vi "Real Time_Master.vi"(4 "File Name":string="none", 8 "Ann Array Params":T1={"Synth Foc?"=FALSE, "Focal Zones"=41, "Switch T/R"=0, "Trans Geometry (mm)"={"Transducer"=0, "Geo Focus"=12.0, "a (radius)"=3.0, "# of rings"=5, "kerf space "=0.1, "Center Freq"=12.0}, "Sub Ap Excite?"=FALSE, "Full Array Scan?"=FALSE, "Xmt/Rcv"={"XMIT"=[TRUE, TRUE, TRUE, TRUE, TRUE], "RCV"=[TRUE, TRUE, TRUE, TRUE, TRUE]}, "PulseSpacing (us)"=0.0, "Xmit Ring"=0, "XMIT CHS"=0, "RCV CHS"=0, "GPU?"=FALSE, "Save TIFF?"=FALSE, "downfactor"=1, "RCV 1CH"=0} {"RCV 1CH" items=["All", "1", "2", "3", "4", "5"]; "Trans Geometry (mm)"."Transducer" items=["6D 12R 40 MHz"=0, "10D 31R 20 MHz"=1, "10D 23R 20 MHz"=2, "6D 23R 40 MHz"=3, "4.5D 10.7R 40 MHz"=4, "9D 23.5R 20 MHz"=5, "9D 25.8R 20MHz"=6, "Enter"=99]; "Switch T/R" min=1 max=5 step=1}, 10 "Motion Settings":T4={"No Motion?"=FALSE, "Motion System"=enum."NI 735x", "Motion Bd ID"=1, "Motion Profile"="SMAC1", "# Axis"=1, "Reverse Z axis?"=TRUE, "SMAC Axis"=0, "scan pair"=enum."y-(x) scan", "RT fps"=6.0, "Steps per mm"=[1000, 1000, 1000, 1000], "Motor Parameters"={"velocity ct/s"=[10000.0, 10000.0, 10000.0, 50000.0], "accel ct/s^2"=[50000.0, 50000.0, 50000.0, 200000.0]}, "One Way Scan"=FALSE, "Reverse One Way Scan"=FALSE, "Global Position (mm)"=[], "Plane"=0, "Distance between\nscan lines (um)"=0.0, "Distance between\nscan planes (um)"=0.0, "number of scan planes"=1, "Total steps in line"=0, "Xtra plane\ndistance  (um)"=100, "Xtra planes "=1, "Add Axis"=FALSE, "overshoot cts"=200, "BKPT Shift"=0, "Scan Start Time (ms)"=0, "ESP VISA"="GPIB::1::INSTR", "3rd Axis"=1, "GL Ref Out"=refnum, "Galil Address"=""} {"3rd Axis" items=["x", "y", "z", "w"]; "Xtra planes" min=1; "Xtra plane\ndistance  (um)" min=0; "Distance between\nscan planes (um)" format="%.2f"; "Distance between\nscan lines (um)" format="%.2f"; "SMAC Axis" items=["None"=0, "Axis 1"=1, "Axis 2"=2, "Axis 3"=3, "Axis 4"=4, "Axis 5"=5, "Axis 6"=6, "Axis 7"=7, "Axis 8"=8, "Vector Space 1"=17, "Vector Space 2"=18, "Vector Space 3"=19, "Vector Space 4"=20]; "Motion Bd ID" min=1 max=32 step=1}, 11 "Digitizer Settings":T8={"Digitizer delay (us) "=0.0, "rf points per line"=2048, "lines per plane"=128, "Samp Rate (Hz)"=100000000.0, "Additional dig delay (us)"=0.0, "Voltage Scale"=0.4, "Pre-Looks"=0, "Offset delay (us)"=0.0, "bits A/D"=8, "Avg Num"=1, "DigTimeOut"=5.0, "Rel Dig Delay"=0.0, "Dig Ch"=0, "LeCroyCluster"={"LeCroy Channels"=[TRUE, FALSE, FALSE, FALSE], "LC read pt offset"=0.0, "Sweep Avg"=FALSE}, "Main Digitizer"=enum."NI Digitizer", "Dig Config"=enum."Single channel", "Digitizer ID Cluster"={"Acqiris/Alazar/SP ID"=[], "NI Instr Handles"=[], "LeCroy VISA"="", "GaGe Handle"={"Handle"=0, "Sample size"=0, "Resolution"=0, "Offset"=0, "Channels"=0, "Boards"=0}, "ATS Ref"="ATS9350", "Acqiris Address"=["PCI::INSTR0"], "ADQRef"=refnum, "adq_cu_ptr"=refnum}, "Trigger Settings"={"Trig Source"=1, "Trig Coupling"=0, "Trig Slope"=0, "Level (mV)"=1500.0}, "Bulk Acq"=FALSE, "Bulk Start Indexes"=[], "Data Ref RF"=refnum, "NI ID/Channel"=[], "Total Dig CH"=1, "Xtra Ann Trig delay (us)"=10.0, "Fix Z Delay?"=FALSE, "One Way Transmission?"=FALSE, "Data Ref Log"=refnum} {"Trigger Settings"."Trig Slope" items=["Positive", "Negative"]; "Trigger Settings"."Level (mV)" format="%.2f"; "Trigger Settings"."Trig Coupling" items=["DC 1 MOhm", "AC 1 MOhm", "DC 50 Ohm", "AC 50 Ohm"]; "Trigger Settings"."Trig Source" items=["Chan 1", "External"]; "Rel Dig Delay" format="%.2f"; "DigTimeOut" format="%.2f"; "Avg Num" min=1; "Offset delay (us)" format="%.2f"; "Additional dig delay (us)" format="%.2f"; "Digitizer delay (us)" format="%.2f"}) -> (0 "Ann Array\nParams Out":T1={"Synth Foc?"=FALSE, "Focal Zones"=41, "Switch T/R"=0, "Trans Geometry (mm)"={"Transducer"=0, "Geo Focus"=12.0, "a (radius)"=3.0, "# of rings"=5, "kerf space "=0.1, "Center Freq"=12.0}, "Sub Ap Excite?"=FALSE, "Full Array Scan?"=FALSE, "Xmt/Rcv"={"XMIT"=[TRUE, TRUE, TRUE, TRUE, TRUE], "RCV"=[TRUE, TRUE, TRUE, TRUE, TRUE]}, "PulseSpacing (us)"=0.0, "Xmit Ring"=0, "XMIT CHS"=0, "RCV CHS"=0, "GPU?"=FALSE, "Save TIFF?"=FALSE, "downfactor"=1, "RCV 1CH"=0} {"RCV 1CH" items=["All", "1", "2", "3", "4", "5"]; "Trans Geometry (mm)"."Transducer" items=["6D 12R 40 MHz"=0, "10D 31R 20 MHz"=1, "10D 23R 20 MHz"=2, "6D 23R 40 MHz"=3, "4.5D 10.7R 40 MHz"=4, "9D 23.5R 20 MHz"=5, "9D 25.8R 20MHz"=6, "Enter"=99]; "Switch T/R" min=1 max=5 step=1}, 2 "Motion Settings Out":T4={"No Motion?"=FALSE, "Motion System"=enum."NI 735x", "Motion Bd ID"=1, "Motion Profile"="SMAC1", "# Axis"=1, "Reverse Z axis?"=TRUE, "SMAC Axis"=0, "scan pair"=enum."y-(x) scan", "RT fps"=6.0, "Steps per mm"=[1000, 1000, 1000, 1000], "Motor Parameters"={"velocity ct/s"=[10000.0, 10000.0, 10000.0, 50000.0], "accel ct/s^2"=[50000.0, 50000.0, 50000.0, 200000.0]}, "One Way Scan"=FALSE, "Reverse One Way Scan"=FALSE, "Global Position (mm)"=[], "Plane"=0, "Distance between\nscan lines (um)"=0.0, "Distance between\nscan planes (um)"=0.0, "number of scan planes"=1, "Total steps in line"=0, "Xtra plane\ndistance  (um)"=100, "Xtra planes "=1, "Add Axis"=FALSE, "overshoot cts"=200, "BKPT Shift"=0, "Scan Start Time (ms)"=0, "ESP VISA"="GPIB::1::INSTR", "3rd Axis"=1, "GL Ref Out"=refnum, "Galil Address"=""} {"3rd Axis" items=["x", "y", "z", "w"]; "Xtra planes" min=1; "Xtra plane\ndistance  (um)" min=0; "Distance between\nscan planes (um)" format="%.2f"; "Distance between\nscan lines (um)" format="%.2f"; "SMAC Axis" items=["None"=0, "Axis 1"=1, "Axis 2"=2, "Axis 3"=3, "Axis 4"=4, "Axis 5"=5, "Axis 6"=6, "Axis 7"=7, "Axis 8"=8, "Vector Space 1"=17, "Vector Space 2"=18, "Vector Space 3"=19, "Vector Space 4"=20]; "Motion Bd ID" min=1 max=32 step=1}, 3 "Digitizer Settings Out":T8={"Digitizer delay (us) "=0.0, "rf points per line"=2048, "lines per plane"=128, "Samp Rate (Hz)"=100000000.0, "Additional dig delay (us)"=0.0, "Voltage Scale"=0.4, "Pre-Looks"=0, "Offset delay (us)"=0.0, "bits A/D"=8, "Avg Num"=1, "DigTimeOut"=5.0, "Rel Dig Delay"=0.0, "Dig Ch"=0, "LeCroyCluster"={"LeCroy Channels"=[TRUE, FALSE, FALSE, FALSE], "LC read pt offset"=0.0, "Sweep Avg"=FALSE}, "Main Digitizer"=enum."NI Digitizer", "Dig Config"=enum."Single channel", "Digitizer ID Cluster"={"Acqiris/Alazar/SP ID"=[], "NI Instr Handles"=[], "LeCroy VISA"="", "GaGe Handle"={"Handle"=0, "Sample size"=0, "Resolution"=0, "Offset"=0, "Channels"=0, "Boards"=0}, "ATS Ref"="ATS9350", "Acqiris Address"=["PCI::INSTR0"], "ADQRef"=refnum, "adq_cu_ptr"=refnum}, "Trigger Settings"={"Trig Source"=1, "Trig Coupling"=0, "Trig Slope"=0, "Level (mV)"=1500.0}, "Bulk Acq"=FALSE, "Bulk Start Indexes"=[], "Data Ref RF"=refnum, "NI ID/Channel"=[], "Total Dig CH"=1, "Xtra Ann Trig delay (us)"=10.0, "Fix Z Delay?"=FALSE, "One Way Transmission?"=FALSE, "Data Ref Log"=refnum} {"Trigger Settings"."Trig Slope" items=["Positive", "Negative"]; "Trigger Settings"."Level (mV)" format="%.2f"; "Trigger Settings"."Trig Coupling" items=["DC 1 MOhm", "AC 1 MOhm", "DC 50 Ohm", "AC 50 Ohm"]; "Trigger Settings"."Trig Source" items=["Chan 1", "External"]; "Rel Dig Delay" format="%.2f"; "DigTimeOut" format="%.2f"; "Avg Num" min=1; "Offset delay (us)" format="%.2f"; "Additional dig delay (us)" format="%.2f"; "Digitizer delay (us)" format="%.2f"})   [LabVIEW 2022 SP3]
uses:
  ScanningControl/Digitizers/-DigitizerRoutines/DigitizerSettings.ctl
  ScanningControl/Digitizers/-DigitizerRoutines/Digitizer.ctl
  ScanningControl/Digitizers/-DigitizerRoutines/DigConfig.ctl
  ScanningControl/Digitizers/-DigitizerRoutines/DigitizerID.ctl
  C:/Windows/System32/ADQAPI_dotNet_helper.dll
  ScanningControl/Motion Controllers/NI_controller/-NI_MotionRoutines/MotionParameters.ctl
  ScanningControl/Motion Controllers/NI_controller/-NI_MotionRoutines/MotionSys.ctl
  ScanningControl/Motion Controllers/-MotionRoutines/ScanAxis.ctl
  ScanningControl/Motion Controllers/-MotionRoutines/3rdAxis.ctl
  Annular Array/-AnnularRoutines/TransGeometry.ctl
  Annular Array/-AnnularRoutines/ArrayGeometry.ctl
  Annular Array/-AnnularRoutines/AnnularArray.ctl
  <vilib>/Utility/miscctls.llb/LVRectTypeDef.ctl
  <vilib>/Utility/miscctls.llb/LVBoundsTypeDef.ctl
  <vilib>/picture/picture.llb/imagedata.ctl
  ScanningControl/Motion Controllers/Galil/Command Menu.ctl
  ScanningControl/Pulsers/PulserGlobals.vi
  ScanningControl/Motion Controllers/-MotionRoutines/MotionGlobals.vi
  <vilib>/Motion/FlexMotion/FunctionsVIs/Trajectory.llb/Load Acceleration/Deceleration.flx
  <vilib>/ptbypt/NI_PtbyPt.lvlib
  <vilib>/Motion/FlexMotion/FunctionsVIs/StartStopMotion.llb/Stop Motion (8 axes).flx
  <vilib>/Motion/FlexMotion/FunctionsVIs/StartStopMotion.llb/Start Motion (8 axes).flx
panel:
  in  "Flip X":bool
  out "No data":bool
  in  "options":T12(tab)
  in  "Focal Zones":i16=41
  in  "Trans Geometry (mm)":T2={"Transducer"=0, "Geo Focus"=12.0, "a (radius)"=3.0, "# of rings"=5, "kerf space "=0.1, "Center Freq"=12.0} {"Transducer" items=["6D 12R 40 MHz"=0, "10D 31R 20 MHz"=1, "10D 23R 20 MHz"=2, "6D 23R 40 MHz"=3, "4.5D 10.7R 40 MHz"=4, "9D 23.5R 20 MHz"=5, "9D 25.8R 20MHz"=6, "Enter"=99]}
  in  "Xmt/Rcv":cluster{"XMIT":bool[], "RCV":bool[]}={"XMIT"=[TRUE, TRUE, TRUE, TRUE, TRUE], "RCV"=[TRUE, TRUE, TRUE, TRUE, TRUE]}
  in  "GPU?":bool
  in  "Daxsonics Settings":T13={"Freq (MHz) "=20, "Amp (V)"=0, "Gain (dB)"=22} {"Freq (MHz)" items=["50"=20, "45"=27, "40"=34, "35"=41, "30"=49, "25"=56, "20"=63, "15"=70]; "Amp (V)" items=["100"=100, "90"=90, "80"=80, "70"=70, "60"=60, "50"=50, "40"=40, "30"=30, "20"=20, "10"=10, "0"=0]; "Gain (dB)" items=["64"=64, "60"=60, "52"=52, "48"=48, "44"=44, "40"=40, "36"=36, "32"=32, "28"=28, "24"=24, "20"=20, "16"=16]}
  in  "RF data Sampling":T14={"Sampling Rate"=100.0, "Ref Delay (ms)"=0.0, "rf points per line"=2048} {"rf points per line" min=1; "Ref Delay (ms)" format="%.2f"}
  in  "Voltage":dbl(ring)=0.2 items=["10 V"=10.0, "4 V"=4.0, "2 V"=2.0, "1 V"=1.0, "400 mV"=0.4, "200 mV"=0.2, "100 mV"=0.1]
  in  "Filter Prams":cluster{"low f":i32, "order":i32, "high F":i32}={"low f"=20, "order"=81, "high F"=65}
  in  "Filter":bool=TRUE
  in  "3D Acq":bool
  in  "Distance between\nplanes (mm)":i32=100 min=0
  in  "number of planes":u16=1
  out "Length of\nall planes (cm)":dbl=128.0 format="%.2f"
  in  "Axis":u16(ring)=1 items=["X Axis"=1, "Y Axis"=2, "Z Axis"=3, "W Axis"=4]
  in  "Position (mm) (Abs)":dbl format="%.3f"
  in  "Axis Tune":enum32{"Axis 1", "Axis 2", "Axis 3", "Axis 4"}(radio)=enum."Axis 2"
  in  "Stop Motor":bool
  in  "Adjust fps (%)":i16(slide)=100 min=0 max=150 scale=0.0..150.0
  in  "Accel":dbl(slide)=11928588.235294117 scale=1000000.0..6500000.0 scale format="%#_6e"
  in  "Inc. Step Size (mm)":dbl=0.5
  in  "LowTime":dbl=0.01
  in  "Gate Length":dbl=0.19 format="%.6f"
  in  "Xtra delay (us)":dbl=1.0
  in  "Aviso Sector":bool
  in  "Motion Parameters":T15={"lines per plane"=128, "Distance between\nscan lines (um)"=100.0, "Frames/s"=2.0, "BKPT Shift"=75, "Overshoot"=200} {"Overshoot" min=0 max=10000; "Distance between\nscan lines (um)" min=0.1 step=0.1; "lines per plane" min=1}
  out "Sat Ct":u8(slide) scale=0.0..400.0
  in  "Pause":bool
  in  "Center":bool
  in  "Scan":bool
  in  "Auto\nScale":bool
  in  "Save Raw":bool
  out "image time (ms)":u32
  out "Image Backlog":i32
  in  "Scale (dB)":cluster{i32, i32}(slide)={-55, 0} scale=0.0..-75.0
  in  "Fill":bool
  in  "1-to-1":bool
  out "InQueue":i32
  out "fps":dbl format="%#.2g"
  in  "N":u8=50 max=50 step=1
  in  "Save Last N EYE":bool
  out "Frame":i32
  in  "EYE CineLoop":bool
  in  "BMP CineLoop":bool
  out "Raw data":dbl[][](graph)
  in  "ExitSendCmd":bool
  # "View"
  # "Data Archiving"
  # "© 2011-2022 WCM"
  # "1-D and 2-D B scan settings"
  # "1-D and 2-D B scan settings"
  # "Daxsonics"
  # "Not working yet and slow."
  # "Cross Axis Motion"
  # "Scan"
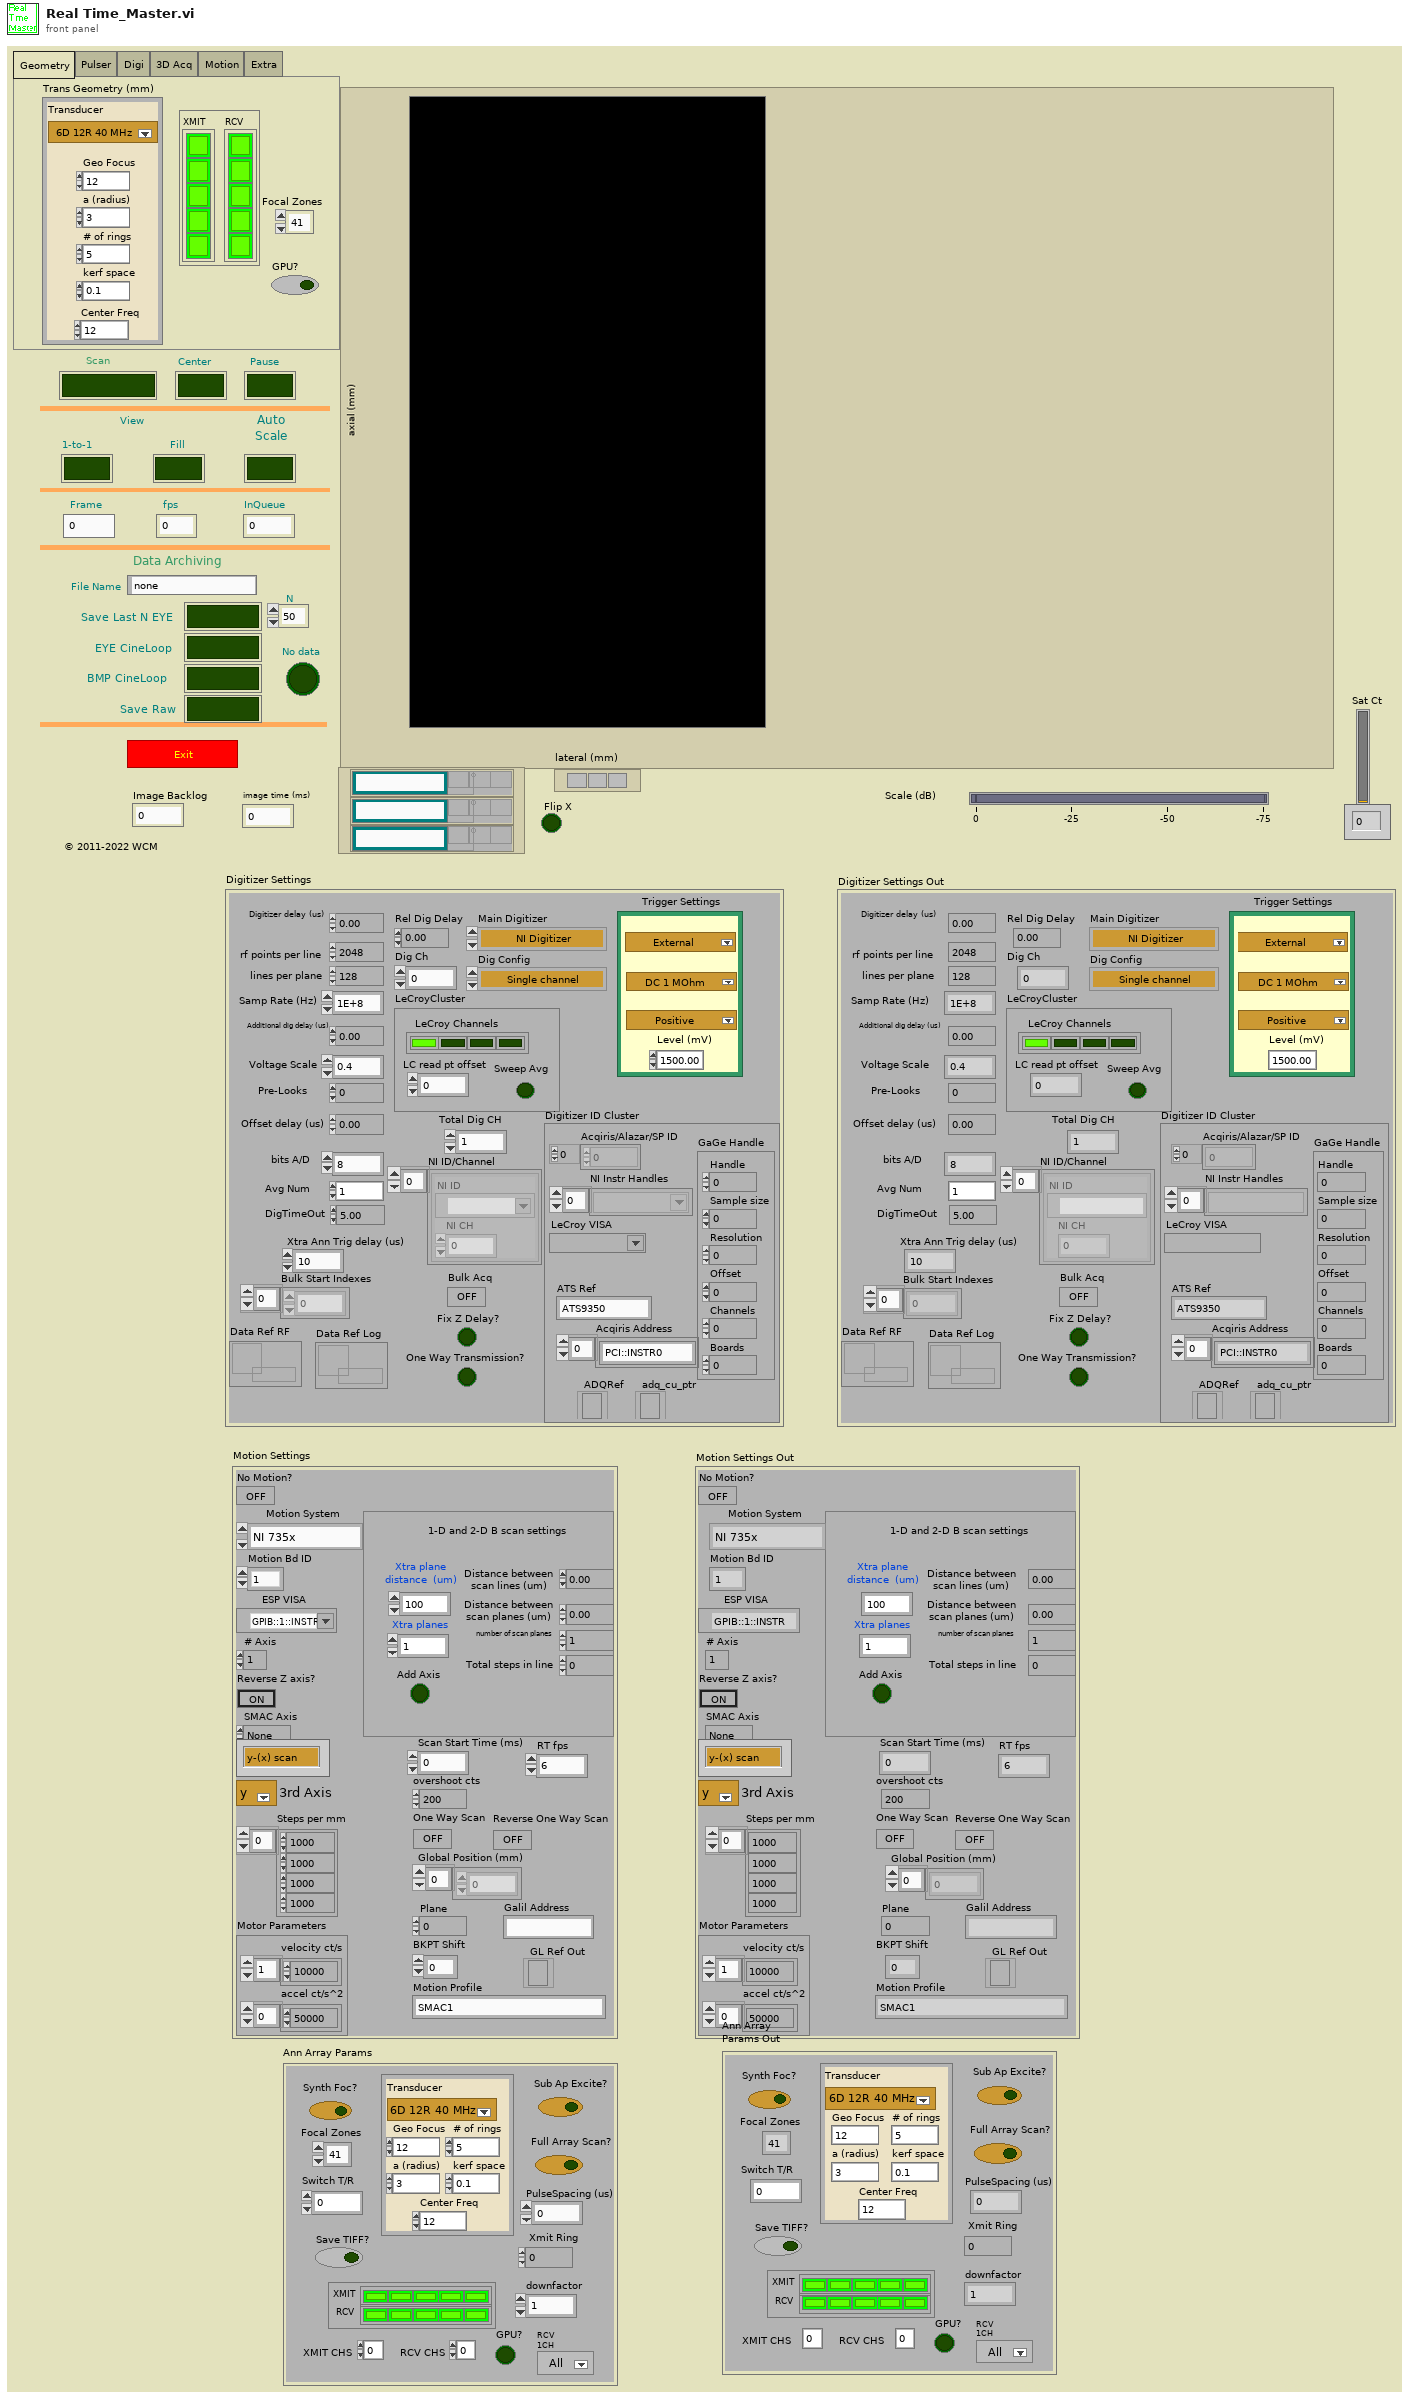
[diagram p1: front panel]
types:
  T1 = typedef "AnnularArray.ctl" = cluster{"Synth Foc?":bool, "Focal Zones":i16, "Switch T/R":i16, "Trans Geometry (mm)":T2, "Sub Ap Excite?":bool, "Full Array Scan?":bool, "Xmt/Rcv":cluster{"XMIT":bool[], "RCV":bool[]}, "PulseSpacing (us)":sgl, "Xmit Ring":i32, "XMIT CHS":u8, "RCV CHS":u8, "GPU?":bool, "Save TIFF?":bool, "downfactor":i32, "RCV 1CH":u16}
  T2 = typedef "TransGeometry.ctl" = cluster{"Transducer":T3, "Geo Focus":dbl, "a (radius)":dbl, "# of rings":i32, "kerf space ":dbl, "Center Freq":dbl}
  T3 = typedef "ArrayGeometry.ctl" = u16
  T4 = typedef "MotionParameters.ctl" = cluster{"No Motion?":bool, "Motion System":T5, "Motion Bd ID":u8, "Motion Profile":string, "# Axis":i8, "Reverse Z axis?":bool, "SMAC Axis":u16, "scan pair":T6, "RT fps":sgl, "Steps per mm":i32[], "Motor Parameters":cluster{"velocity ct/s":dbl[], "accel ct/s^2":dbl[]}, "One Way Scan":bool, "Reverse One Way Scan":bool, "Global Position (mm)":dbl[], "Plane":i32, "Distance between\nscan lines (um)":sgl, "Distance between\nscan planes (um)":sgl, "number of scan planes":i32, "Total steps in line":i32, "Xtra plane\ndistance  (um)":i32, "Xtra planes ":i32, "Add Axis":bool, "overshoot cts":i32, "BKPT Shift":i32, "Scan Start Time (ms)":u32, "ESP VISA":refnum<visa-resource-name>, "3rd Axis":T7, "GL Ref Out":refnum<k7>, "Galil Address":string}
  T5 = typedef "MotionSys.ctl" = enum16{"MM3000", "NI 735x", "Newport ESP", "No Motion Card", "Galil"}
  T6 = typedef "ScanAxis.ctl" = enum16{"y-(x) scan", "x-(y) scan", "z-(x) scan", "z-(y) scan", "y-(z) scan", "x-(z) scan", "w-(x) scan", "w-(y) scan", "w-(z) scan", "x-(w) scan", "y-(w) scan", "z-(w) scan"}
  T7 = typedef "3rdAxis.ctl" = u16
  T8 = typedef "DigitizerSettings.ctl" = cluster{"Digitizer delay (us) ":dbl, "rf points per line":i32, "lines per plane":i32, "Samp Rate (Hz)":dbl, "Additional dig delay (us)":dbl, "Voltage Scale":dbl, "Pre-Looks":i32, "Offset delay (us)":dbl, "bits A/D":i8, "Avg Num":i32, "DigTimeOut":sgl, "Rel Dig Delay":sgl, "Dig Ch":i32, "LeCroyCluster":cluster{"LeCroy Channels":bool[], "LC read pt offset":dbl, "Sweep Avg":bool}, "Main Digitizer":T9, "Dig Config":T10, "Digitizer ID Cluster":T11, "Trigger Settings":cluster{"Trig Source":u16, "Trig Coupling":u16, "Trig Slope":u16, "Level (mV)":dbl}, "Bulk Acq":bool, "Bulk Start Indexes":i32[], "Data Ref RF":refnum<data-value>, "NI ID/Channel":cluster{"NI ID":refnum<k15>, "NI CH":i32}[], "Total Dig CH":i32, "Xtra Ann Trig delay (us)":dbl, "Fix Z Delay?":bool, "One Way Transmission?":bool, "Data Ref Log":refnum<data-value>}
  T9 = typedef "Digitizer.ctl" = enum16{"Acqiris Digitizer", "NI Digitizer", "LeCroy", "GaGe", "AlazarTech", "No Digitizer", "Teledyne"}
  T10 = typedef "DigConfig.ctl" = enum16{"Single channel", "2 Chans w/ 2 Acqiris", "2 Chans w/ 1 Acqiris", "5-CH Pulser New", "5-CH pulser w/ ann array", "5-pass style ann array", "Empty"}
  T11 = typedef "DigitizerID.ctl" = cluster{"Acqiris/Alazar/SP ID":u32[], "NI Instr Handles":refnum<k15>[], "LeCroy VISA":refnum<visa-resource-name>, "GaGe Handle":cluster{"Handle":u32, "Sample size":u32, "Resolution":i32, "Offset":i32, "Channels":u32, "Boards":u32}, "ATS Ref":string, "Acqiris Address":string[], "ADQRef":refnum<k24>, "adq_cu_ptr":refnum<k24>}
  T12 = enum32{"Geometry", "Pulser", "Digi", "3D Acq", "Motion", "Extra"}
  T13 = cluster{"Freq (MHz) ":u16, "Amp (V)":u16, "Gain (dB)":u16}
  T14 = cluster{"Sampling Rate":dbl, "Ref Delay (ms)":dbl, "rf points per line":i32}
  T15 = cluster{"lines per plane":u16, "Distance between\nscan lines (um)":sgl, "Frames/s":sgl, "BKPT Shift":i32, "Overshoot":i32}
  T16 = typedef "LVBoundsTypeDef.ctl" = cluster{"Width":u32, "Height":u32}
  T17 = typedef "LVRectTypeDef.ctl" = cluster{"Left":i16, "Top":i16, "Right":i16, "Bottom":i16}
  T18 = typedef "pulser.ctl" = enum16{"Pan 5900", "Daxsonics", "Agilent 33xxx", "UTEX", "JSR", "WMC Mono-Cycle", "No Pulser", "NYU AVTECH", "Tabor W1281A", "Pan 5800", "Unlisted", "Tabor WX2182B"}
  T19 = typedef "location.ctl" = enum16{"Automatic", "WCM Main", "Hawaii", "Columbia MM3000", "Columbia  NI System", "NYU", "RRI 2", "UHI Allen", "CUMC RT", "Chiba", "Stony Brook", "WCM Microscopy", "WCM Aeoretch", "WCM Optics Lab", "WCM Main 2Axis", "WCM Rotation", "WCM SAM SMAC", "SERI GP"}
  T20 = cluster{"DataBufferQ":refnum<queue>, "LastNQ":refnum<queue>, "LastNBMPQ":refnum<queue>, "SaveRawN":refnum<notifier>, "StopN":refnum<notifier>}
  T21 = typedef "imagedata.ctl" = cluster{"image type":i32, "image depth":i32, "image":u8[], "mask":u8[], "colors":u32[], "Rectangle":cluster{"left":i16, "top":i16, "right":i16, "bottom":i16}}
  T22 = cluster{"gain":dbl, bool, "wfm":i16[][], i32, bool}
  T23 = enum16{"Absolute Position", "Relative Position", "Velocity", "Relative to Cap Pos", "Modulus Position", "Absolute Contouring", "Relative Contouring"}
  T24 = cluster{"Voltage Scale":dbl, "Offset":dbl, "Coupling":u16}
  T25 = enum16{"Home", "Index", "Center", "Forward Limit", "Reverse Limit", "Run Sequence"}
  T26 = typedef "Command Menu.ctl" = enum16{"CommandPassThrough", "Abort Motion", "Define Pos", "Velocity", "Acceleration", "Deceleration", "Position Rel", "Postion Abs", "Begin Move", "After Move", "Home", "KI", "KD", "KP", "IL", "Config I/O", "Set Bit", "Clear Bit", "Motor Off", "Moto On", "Status", "Execute", "Halt Execute", "HX Status", "Tell Velocity", "Check Motion", "BreakPoint", "Tell Position", "Current Code Line", "Tell Switches", "OC Force On", "OC Off", "Pos Soft Limit", "Rev Soft Limit"}
  T27 = typedef "LVStringsAndValuesArrayTypeDef_DBL.ctl" = cluster{"String":string, "Value":dbl}[]
  T28 = cluster{"Samp Rate (Hz)":dbl, "Digitizer delay (us) ":dbl, "rf points per line":i32}
  T29 = typedef "LVStringsAndValuesArrayTypeDef_U16.ctl" = cluster{"String":string, "Value":u16}[]
  T30 = typedef "Dax_Control_Cluster.ctl" = cluster{"Freq (MHz) ":u16, "Voltage (V)":u16, "Gain (dB)":u16}
  T31 = cluster{"Axis scaling Params":cluster{"X right":dbl, "X left":dbl, "Y low":dbl, "Y high":dbl}, "x scaled":dbl[][], "y scaled":dbl[][], "scales":cluster{"inc x (mm)":dbl, "inc y (mm)":dbl}, "Array":dbl[][], "pixels in x":i16, "pixels in y":i16}
  T32 = cluster{"FIR Windowed Coefficients":dbl[], "Filter Prams":cluster{"low f":i32, "order":i32, "high F":i32}}
  T33 = cluster{"gain":dbl, bool, "wfm":i16[][], "max queue size (-1, unlimited)":i32, "Time Out":bool}
  T34 = typedef "eventvkey.ctl" = enum16{"ASCII", "Enter", "Return", "Shift", "Ctrl", "Alt", "Cmd", "Opt", "Caps", "NumLock", "Clear", "Break", "Up", "Down", "Left", "Right", "Insert", "Delete", "Home", "End", "PageUp", "PageDown", "Escape", "Help", "Pause", "ScrollLock", "F1", "F2", "F3", "F4", "F5", "F6", "F7", "F8", "F9", "F10", "F11", "F12", "F13", "F14", "F15", "F16", "F17", "F18", "F19", "F20", "F21", "F22", "F23", "F24", "Play", "VolumeUp", "VolumeDown", "Mute", "Two Byte Char"}
  T35 = cluster{"Shift":bool, "Ctrl":bool, "Alt":bool, "Cmd":bool, "Opt":bool}
  T36 = typedef "Resource Out (Enum).flx" = u16
  T37 = typedef "Bd Id Out" = u8
  T38 = cluster{"Y Scale Offset":dbl, "Y Scale Multi":dbl, "X Scale Offset":dbl, "X Scale Multi":dbl, "Gate Distance":dbl}
  T39 = typedef "AxisOrVectorSpaceControl To Control.flx" = u16
  T40 = typedef "LVRangeTypeDef.ctl" = cluster{"Minimum":dbl, "Maximum":dbl, "Increment":dbl, "Minor Increment":dbl, "Start":dbl}
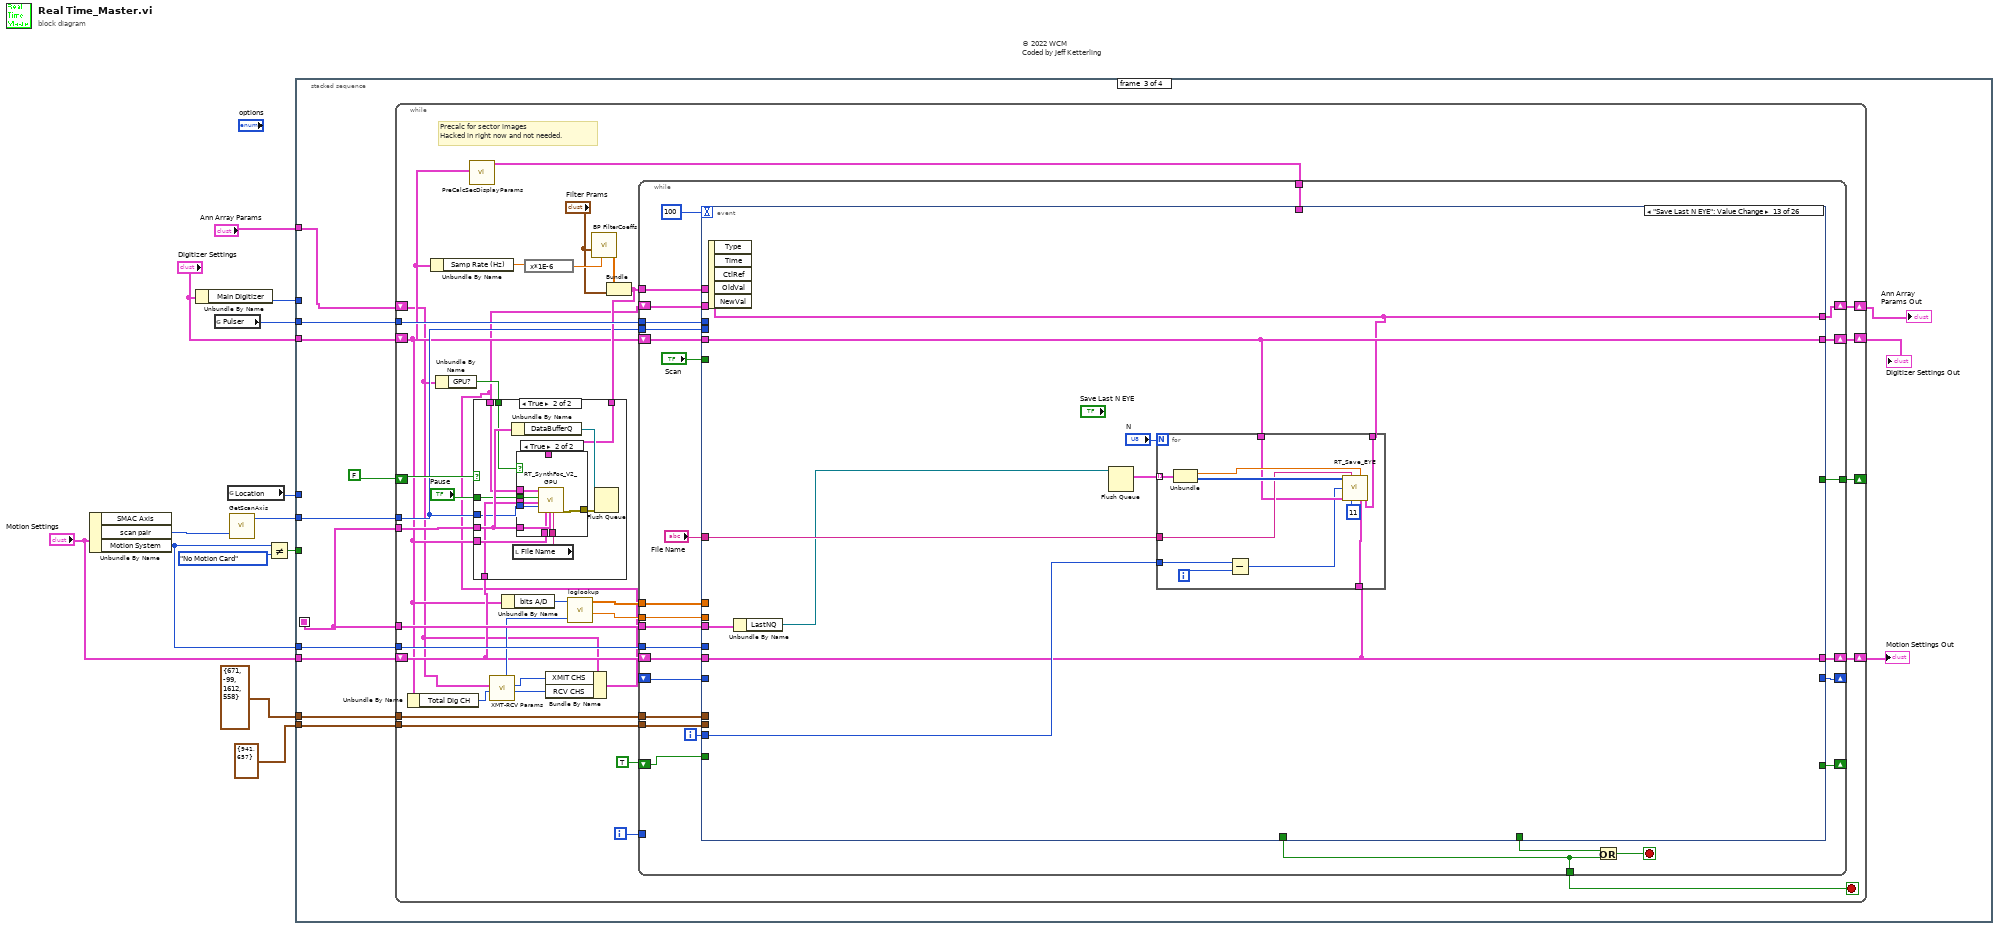
[diagram p0: block diagram]
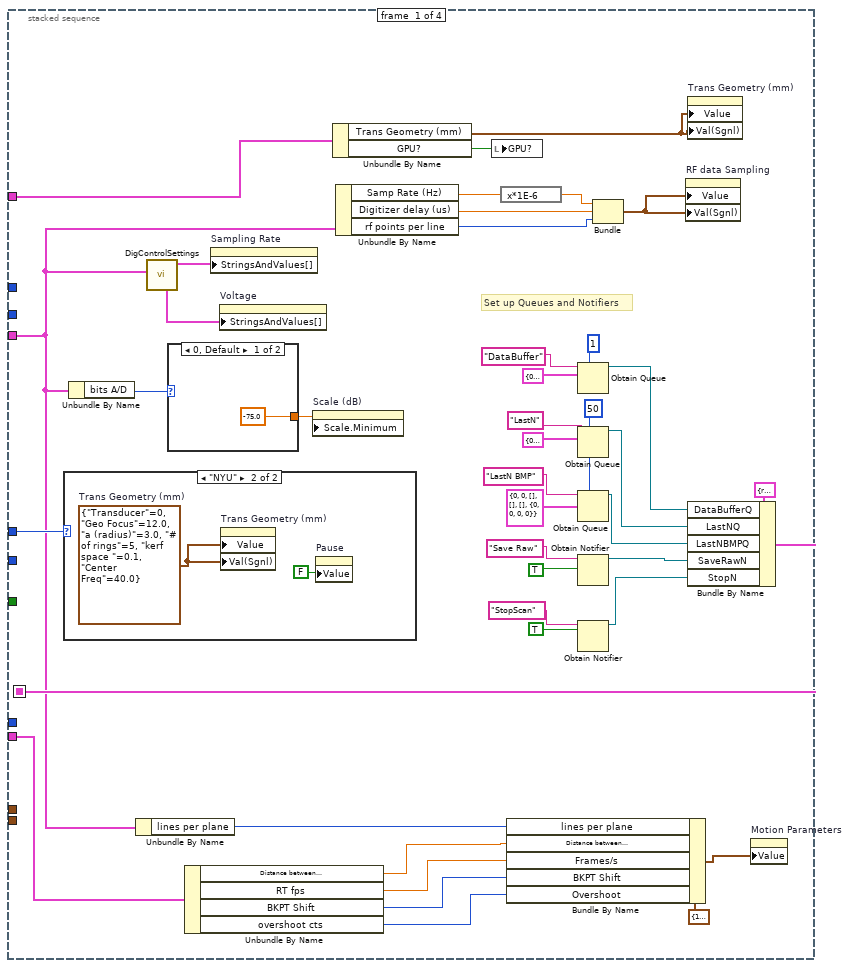
[diagram p2: hidden frame]
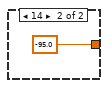
[diagram p4: hidden frame]
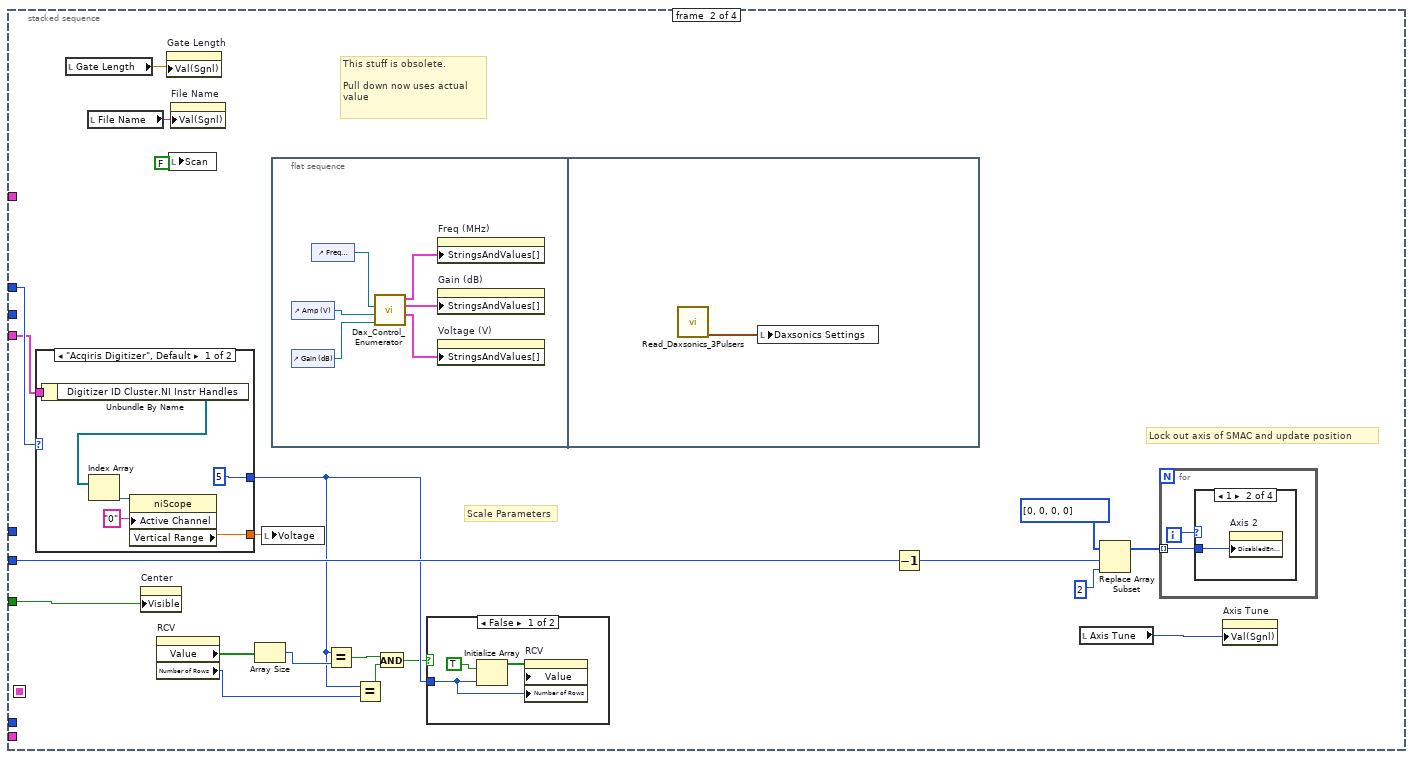
[diagram p5: hidden frame]
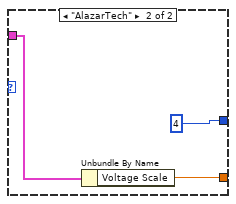
[diagram p7: hidden frame]
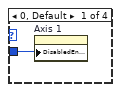
[diagram p8: hidden frame]
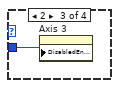
[diagram p9: hidden frame]
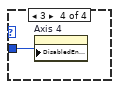
[diagram p10: hidden frame]
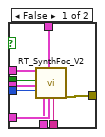
[diagram p12: hidden frame]
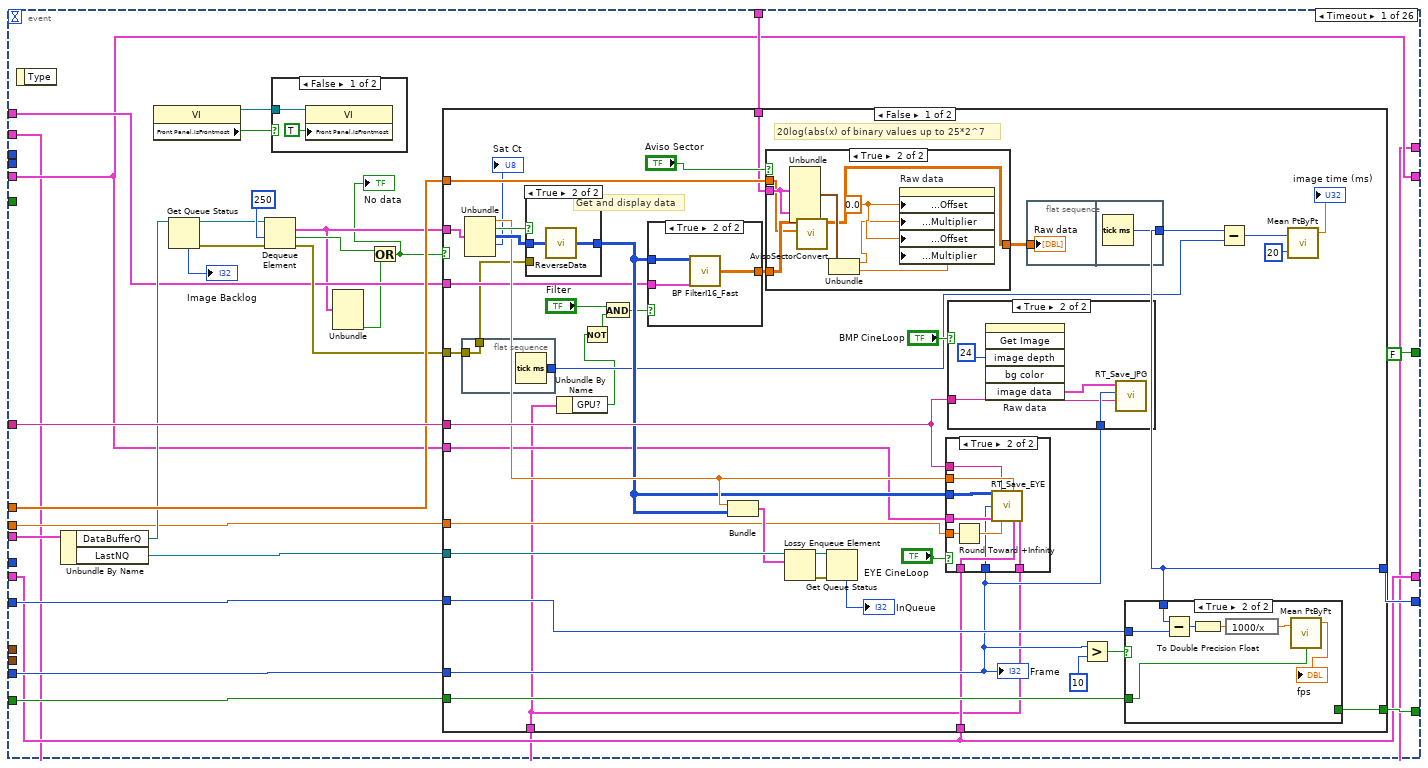
[diagram p13: hidden frame]
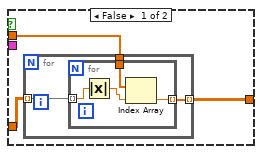
[diagram p15: hidden frame]
diagram:
  # "© 2022 WCM\nCoded by Jeff Ketterling"
  n1 = Unbundle By Name("Motion Settings") -> ("scan pair"=w6:T6, "Motion System"=w7:T5)  [unwired: 1 out]
  n2 = Unbundle By Name("Digitizer Settings") -> ("Main Digitizer"=w9:T9)
  n3 = global read "PulserGlobals.vi" "Pulser"() -> (w4:T18)
  n4 = global read "MotionGlobals.vi" "Location"() -> (w2:T19)
  n5 = call "GetScanAxis.vi"("scan pair"=w6) -> ("Axis 1"=w5:i32)  [unwired: 1 in, 2 out]
  n6 = Not Equal?(x=w7, y=MotionSys."No Motion Card" ("Motion System")) -> (x != y?=w11:bool)
  n7 = stacked-sequence {
    seq-local: [w38 _ _ _] -> [_ _ w112 w857]
    tunnel: T16 {"Width"=941, "Height"=657} ("Plot Area:Size") -> [_ _ w115 _]
    tunnel: T17 {"Left"=671, "Top"=-99, "Right"=1612, "Bottom"=558} ("Plot Area Bounds") -> [_ _ w114 _]
    tunnel: w5 -> [_ w72 w113 _]
    tunnel: w11 -> [_ w76 _ _]
    tunnel: w7 -> [_ _ w111 _]
    tunnel: w4 -> [_ _ w110 _]
    tunnel: w9 -> [_ w68 _ _]
    tunnel: "Digitizer Settings" -> [w14 w59 w109 _]
    tunnel: "Motion Settings" -> [w23 _ w107 _]
    tunnel: w2 -> [w26 _ _ _]
    tunnel: "Ann Array Params" -> [w24 _ w104 _]
    frame #0 {
      w31 = 50 ("max queue size (-1, unlimited)")
      # "Set up Queues and Notifiers"
      n8 = case shown="\"NYU\"" w26 {
        frame "WCM Main", Default {
        }
        frame "NYU" {
          w55 = T2 {"Transducer"=0, "Geo Focus"=12.0, "a (radius)"=3.0, "# of rings"=5, "kerf space "=0.1, "Center Freq"=40.0}  # Trans Geometry (mm)
          n9 = property on="Trans Geometry (mm)" class="Clust (strict)"("Value"=w55, "Val(Sgnl)"=w55) -> ()  [unwired: 2 in, 2 out]
          n10 = property on="Pause" class="Bool (strict)"("Value"=FALSE ("Pause")) -> ()  [unwired: 2 in, 2 out]
        }
      }
      n11 = Unbundle By Name(w14) -> ("bits A/D"=w27:i8)
      n12 = Unbundle By Name(w14) -> ("lines per plane"=w22:i32)
      n13 = call "DigControlSettings.vi"("Digitizer Settings"=w14) -> ("Sampling Rates"=w34:T27, "Voltage Scale"=w33:T27)  [unwired: 6 in, 3 out]
      n14 = case shown="0, Default" w27 {
        tunnel: [-75.0 ("Scale.Range:Maximum") -95.0 ("Scale.Range:Maximum")] -> w32
        frame 0, Default {
        }
        frame 14 {
        }
      }
      n15 = Unbundle By Name(w23) -> ("Distance between\nscan lines (um)"=w21:sgl, "RT fps"=w20:sgl, "BKPT Shift"=w19:i32, "overshoot cts"=w18:i32)
      n16 = property on="Sampling Rate" class="Ring (strict)"("StringsAndValues[]"=w34) -> ()  [unwired: 2 in, 2 out]
      n17 = property on="Voltage" class="Ring (strict)"("StringsAndValues[]"=w33) -> ()  [unwired: 2 in, 2 out]
      n18 = property on="Scale (dB)" class="Slide (strict)"("Scale.Minimum"=w32) -> ()  [unwired: 2 in, 2 out]
      n19 = Unbundle By Name(w24) -> ("Trans Geometry (mm)"=w15:T2, "GPU?"=w25:bool)
      n20 = Unbundle By Name(w14) -> ("Samp Rate (Hz)"=w30:dbl, "Digitizer delay (us)"=w29:dbl, "rf points per line"=w28:i32)
      n21 = local write "GPU?"(w25) -> ()
      n22 = expression code="x*1E-6"(w30) -> (w35:dbl)
      n23 = Bundle By Name(cluster=T15 {"lines per plane"=128, "Distance between\nscan lines (um)"=100.0, "Frames/s"=2.0, "BKPT Shift"=75, "Overshoot"=200} ("Motion Parameters"), "lines per plane"=w22, "Distance between\nscan lines (um)"=w21, "Frames/s"=w20, "BKPT Shift"=w19, "Overshoot"=w18) -> (w16:T15)
      n24 = Obtain Queue(max queue size (-1, unlimited)=1, name (unnamed)="DataBuffer", element data type=T22 {"gain"=0.0, TRUE, "wfm"=[], 0, TRUE}) -> (queue out=w41:refnum<queue>)  [unwired: 2 in, 2 out]
      n25 = Obtain Queue ("LastN")(max queue size (-1, unlimited)=w31, name (unnamed)="LastN", element data type=cluster{"gain":dbl, "wfm":i16[][]} {"gain"=0.0, "wfm"=[]}) -> (queue out=w42:refnum<queue>)  [unwired: 2 in, 2 out]
      n26 = Obtain Queue ("LastNBMP")(max queue size (-1, unlimited)=w31, name (unnamed)="LastN BMP", element data type=T21 {"image type"=0, "image depth"=0, "image"=[], "mask"=[], "colors"=[], "Rectangle"={"left"=0, "top"=0, "right"=0, "bottom"=0}} ("Image Data")) -> (queue out=w40:refnum<queue>)  [unwired: 2 in, 2 out]
      n27 = Obtain Notifier ("Raw eye")(name (unnamed)="Save Raw", notification data type=TRUE) -> (notifier out=w43:refnum<notifier>)  [unwired: 2 in, 2 out]
      n28 = Obtain Notifier ("Stop Scan")(name (unnamed)="StopScan", notification data type=TRUE) -> (notifier out=w39:refnum<notifier>)  [unwired: 2 in, 2 out]
      n29 = Bundle("Samp Rate (Hz)"=w35, "Digitizer delay (us)"=w29, "rf points per line"=w28) -> (w36:T28)  [unwired: 1 in]
      n30 = property on="RF data Sampling" class="Clust (strict)"("Value"=w36, "Val(Sgnl)"=w36) -> ()  [unwired: 2 in, 2 out]
      n31 = property on="Trans Geometry (mm)" class="Clust (strict)"("Value"=w15, "Val(Sgnl)"=w15) -> ()  [unwired: 2 in, 2 out]
      n32 = Bundle By Name(cluster=T20 {"DataBufferQ"=refnum, "LastNQ"=refnum, "LastNBMPQ"=refnum, "SaveRawN"=refnum, "StopN"=refnum} ("Qs and Notis"), "DataBufferQ"=w41, "LastNQ"=w42, "LastNBMPQ"=w40, "SaveRawN"=w43, "StopN"=w39) -> (w38:T20)
      n33 = property on="Motion Parameters" class="Clust (strict)"("Value"=w16) -> ()  [unwired: 2 in, 2 out]
    }
    frame #1 {
      # "This stuff is obsolete.\n\nPull down now uses actual value"
      # "Lock out axis of SMAC and update position"
      # "Scale Parameters"
      n34 = case shown="\"Acqiris Digitizer\", Default" w68 {
        tunnel: [w85 w88] -> w69
        tunnel: [5 4] -> w65
        tunnel: w59 -> [w82 w89]
        frame "Acqiris Digitizer", Default {
          n35 = Unbundle By Name(w82) -> ("Digitizer ID Cluster.NI Instr Handles"=w83:refnum<k15>[])
          n36 = Index Array(array=w83) -> (element=w87:refnum<k15>)  [unwired: 1 in]
          n37 = property class="niScope"(reference=w87, "Active Channel"="0") -> ("Vertical Range"=w85:dbl)  [unwired: 1 in, 2 out]
        }
        frame "AlazarTech" {
          n38 = Unbundle By Name(w89) -> ("Voltage Scale"=w88:dbl)
        }
      }
      n39 = local read "Gate Length"() -> (w60:dbl)
      n40 = local read "File Name"() -> (w77:string)
      n41 = property on="Center" class="Bool"("Visible"=w76) -> ()  [unwired: 2 in, 2 out]
      n42 = property on="RCV" class="Arr (strict)"() -> ("Value"=w67:bool[], "Number of Rows"=w64:u32)  [unwired: 2 in, 2 out]
      n43 = property on="Gate Length" class="DigNum (strict)"("Val(Sgnl)"=w60) -> ()  [unwired: 2 in, 2 out]
      n44 = local write "Scan"(FALSE ("go")) -> ()
      n45 = property on="File Name" class="Str"("Val(Sgnl)"=w77) -> ()  [unwired: 2 in, 2 out]
      n46 = Array Size(array=w67) -> (size(s)=w66:i32)
      n47 = local write "Voltage"(w69) -> ()
      n48 = flat-sequence {
        frame #0 {
          n49 = control-ref of="Amp (V)"() -> (w92:refnum<vi>)
          n50 = control-ref of="Gain (dB)"() -> (w91:refnum<vi>)
          n51 = control-ref of="Freq (MHz)"() -> (w93:refnum<vi>)
          n52 = call "Dax_Control_Enumerator.vi"("Gain (dB) Ref"=w91, "Voltage (V) Ref"=w92, "Freq (MHz) Ref"=w93) -> ("Voltage"=w94:T29, "Gain"=w95:T29, "Freq"=w96:T29)  [unwired: 6 in]
          n53 = property on="Freq (MHz)" class="Ring (strict)"("StringsAndValues[]"=w96) -> ()  [unwired: 2 in, 2 out]
          n54 = property on="Gain (dB)" class="Ring (strict)"("StringsAndValues[]"=w95) -> ()  [unwired: 2 in, 2 out]
          n55 = property on="Voltage (V)" class="Ring (strict)"("StringsAndValues[]"=w94) -> ()  [unwired: 2 in, 2 out]
        }
        frame #1 {
          n56 = call "Read_Daxsonics_3Pulsers.vi"() -> ("Dax Values"=w97:T30)  [unwired: 5 in, 6 out]
          n57 = local write "Daxsonics Settings"(w97) -> ()
        }
      }
      n58 = Equal?(x=w65, y=w66) -> (x = y?=w63:bool)
      n59 = Equal?(x=w65, y=w64) -> (x = y?=w62:bool)
      n60 = And(x=w63, y=w62) -> (x .and. y?=w61:bool)
      n61 = case shown="False" w61 {
        tunnel: w65 -> [w79 _]
        frame False {
          n62 = Initialize Array(TRUE, w79) -> (w80:bool[])
          n63 = property on="RCV" class="Arr (strict)"("Value"=w80, "Number of Rows"=w79) -> ()  [unwired: 2 in, 2 out]
        }
        frame True {
        }
      }
      n64 = Decrement(x=w72) -> (x-1=w70:i32)
      n65 = local read "Axis Tune"() -> (w71:enum32{"Axis 1", "Axis 2", "Axis 3", "Axis 4"})
      n66 = Replace Array Subset(array=i32[] [0, 0, 0, 0], new element=2 ("new element/subarray"), index=w70) -> (w73:i32[])
      n67 = for {
        tunnel: w73 -> [w98] mode=indexing
        i -> [w99]
        n68 = case shown="1" w99 {
          tunnel: w98 -> [w100 w101 w102 w103]
          frame 0, Default {
            n69 = property on="Axis 1" class="Bool (strict)"("DisabledEnum"=w100) -> ()  [unwired: 2 in, 2 out]
          }
          frame 1 {
            n70 = property on="Axis 2" class="Bool (strict)"("DisabledEnum"=w101) -> ()  [unwired: 2 in, 2 out]
          }
          frame 2 {
            n71 = property on="Axis 3" class="Bool (strict)"("DisabledEnum"=w102) -> ()  [unwired: 2 in, 2 out]
          }
          frame 3 {
            n72 = property on="Axis 4" class="Bool (strict)"("DisabledEnum"=w103) -> ()  [unwired: 2 in, 2 out]
          }
        }
      }
      n73 = property on="Axis Tune" class="RadioBtnsControl (strict)"("Val(Sgnl)"=w71) -> ()  [unwired: 2 in, 2 out]
    }
    frame #2 {
      n74 = while {
        shift-right: [w149] -> _
        shift-left: FALSE ("go") -> [w150]
        tunnel: w115 -> [w146]
        tunnel: w114 -> [w145]
        tunnel: w113 -> [w125]
        tunnel: w112 -> [w142]
        tunnel: w112 -> [w141]
        tunnel: w111 -> [w138]
        tunnel: w110 -> [w137]
        shift-right: [w130] -> w108
        shift-left: w109 -> [w124]
        shift-right: [w126] -> w106
        shift-left: w107 -> [w127]
        shift-right: [w120] -> w105
        shift-left: w104 -> [w118]
        i -> [w147]
        stop <- w148 stop-if-true
        # "Precalc for sector images\nHacked in right now and not needed."
        n75 = Unbundle By Name(w124) -> ("Total Dig CH"=w123:i32)
        n76 = Unbundle By Name(w124) -> ("Samp Rate (Hz)"=w131:dbl)
        n77 = Unbundle By Name(w118) -> ("GPU?"=w119:bool)
        n78 = call "PreCalcSecDisplayParams.vi"("Digitizer Settings"=w124) -> ("Cluster out"=w128:T31)  [unwired: 10 in]
        n79 = call "XMT-RCV Params.vi"("Dig Channels"=w123, "Ann Array Params"=w118) -> ("# RCV"=w121:i16, "# XMIT"=w122:i16, "virtual T/R count"=w133:i16)  [unwired: 4 in, 3 out]
        n80 = Unbundle By Name(w124) -> ("bits A/D"=w129:i8)
        n81 = expression code="x*1E-6"(w131) -> (w140:dbl)
        n82 = Bundle By Name(cluster=w118, "XMIT CHS"=w122, "RCV CHS"=w121) -> (w117:T1)
        n83 = call "loglookup.vi"("A/D bits"=w129, "virtual T/R Pairs"=w133) -> ("Log Lookup"=w143:sgl[], "BFormed Bits"=w132:dbl)  [unwired: 1 in, 2 out]
        n84 = call "BP FilterCoeffs.vi"("sample rate MHz"=w140, "Filter Prams"="Filter Prams") -> ("FIR Windowed Coefficients"=w136:dbl[])  [unwired: 4 in]
        n85 = Bundle("FIR Windowed Coefficients"=w136, "Filter Prams"="Filter Prams") -> (w134:T32)  [unwired: 1 in]
        n86 = case shown="True" w150 {
          tunnel: w142 -> [_ w160]
          tunnel: "Pause" -> [_ w157]
          tunnel: w134 -> [_ w156]
          tunnel: w124 -> [_ w155]
          tunnel: w127 -> [_ w154]
          tunnel: w125 -> [_ w153]
          tunnel: w117 -> [_ w152]
          tunnel: w119 -> [_ w151]
          frame False {
          }
          frame True {
            n87 = Unbundle By Name(w160) -> ("DataBufferQ"=w159:refnum<queue>)
            n88 = local read "File Name"() -> (w158:string)
            n89 = case shown="True" w151 {
              tunnel: [w170 w178] -> w161
              tunnel: w160 -> [w169 w177]
              tunnel: w158 -> [w168 w176]
              tunnel: w157 -> [w167 w175]
              tunnel: w156 -> [w166 _]
              tunnel: w155 -> [w165 w174]
              tunnel: w154 -> [w164 w173]
              tunnel: w153 -> [w163 w172]
              tunnel: w152 -> [w162 w171]
              frame False {
                n90 = call "RT_SynthFoc_V2.vi"("Ann Array Params"=w162, "Pause?"=w167, "Motion Settings"=w164, "Scan Axis"=w163, "Digitizer Settings"=w165, "Filter"=w166, "Qs and Notis"=w169, "Raw Name"=w168) -> ("error out"=w170:errorcluster)  [unwired: 10 in, 1 out]
              }
              frame True {
                n91 = call "RT_SynthFoc_V2_GPU.vi"("Ann Array Params"=w171, "Pause?"=w175, "Motion Settings"=w173, "Scan Axis"=w172, "Digitizer Settings"=w174, "Qs and Notis"=w177, "Raw Name"=w176) -> ("error out"=w178:errorcluster)  [unwired: 11 in, 1 out]
              }
            }
            n92 = Flush Queue(queue=w159, error in (no error)=w161) -> ()  [unwired: 3 out]
          }
        }
        n93 = while {
          tunnel: [w203] -> w149
          tunnel: [w200] -> w148
          tunnel: w147 -> [_]
          shift-right: [w199] -> _
          shift-left: _ -> [w198]
          tunnel: w146 -> [w197]
          tunnel: w145 -> [w196]
          tunnel: w125 -> [w195]
          shift-right: [w193] -> _
          shift-left: TRUE -> [w194]
          tunnel: w143 -> [w192]
          tunnel: w141 -> [w190]
          tunnel: w138 -> [w189]
          tunnel: w137 -> [w188]
          tunnel: w134 -> [w187]
          tunnel: w132 -> [w186]
          tunnel: w128 -> [w185]
          shift-right: [w183] -> w130
          shift-left: w124 -> [w184]
          shift-right: [w181] -> w126
          shift-left: w127 -> [w182]
          shift-right: [w179] -> w120
          shift-left: w117 -> [w180]
          i -> [w206]
          stop <- w201 stop-if-true
          n94 = event shown="[12] \"Save Last N EYE\": Value Change" {
            selector: _ -> [_ _ _ _ _ _ _ _ _ _ _ _ _ _ _ _ _ _ _ _ _ _ _ _ _ _]
            dyn-events: _ -> [_ _ _ _ _ _ _ _ _ _ _ _ _ _ _ _ _ _ _ _ _ _ _ _ _ _]
            timeout: 100 -> [_ _ _ _ _ _ _ _ _ _ _ _ _ _ _ _ _ _ _ _ _ _ _ _ _ _]
            tunnel: w206 -> [w229 _ w357 _ _ _ _ _ _ _ _ _ w639 _ _ _ _ _ _ _ _ _ _ _ _ _]
            tunnel: "File Name" -> [w234 _ w377 _ _ _ _ _ _ _ _ _ w638 _ _ _ _ _ _ _ _ _ _ _ _ _]
            tunnel: [FALSE ("go") _ FALSE ("go") _ w484 w503 w528 w542 w597 _ _ _ _ _ _ _ _ _ _ _ _ _ _ _ _ _] -> w203
            tunnel: [_ _ _ _ w484 w503 w528 w542 w597 _ _ _ _ _ _ _ _ _ _ _ _ _ _ _ _ _] -> w202
            tunnel: [_ _ _ _ _ _ _ _ _ _ "ExitSendCmd" _ _ _ _ _ _ _ _ _ _ _ _ _ _ _] -> w200
            tunnel: [w231 _ _ _ _ _ _ _ _ _ _ _ _ _ _ _ _ _ _ _ _ _ _ _ _ _] -> w199
            tunnel: w198 -> [w230 _ _ _ _ _ _ _ _ _ _ _ _ _ _ _ _ _ _ _ _ _ _ _ _ _]
            tunnel: w197 -> [_ _ _ _ _ _ _ _ _ _ _ _ _ _ w663 _ _ _ _ _ _ _ _ _ _ _]
            tunnel: w196 -> [_ _ _ _ _ _ _ _ _ _ _ _ _ _ w662 _ _ w725 _ _ _ _ _ _ _ _]
            tunnel: w195 -> [_ _ _ _ _ _ _ _ w583 _ _ _ _ _ _ _ w699 _ _ _ w741 w752 _ w775 _ _]
            tunnel: w194 -> [w228 _ _ _ _ _ _ _ _ _ _ _ _ _ _ _ _ _ _ _ _ _ _ _ _ _]
            tunnel: [w227 _ _ _ _ _ _ _ _ _ _ _ _ _ _ _ _ _ _ _ _ _ _ _ _ _] -> w193
            tunnel: w192 -> [w226 _ w375 _ _ _ _ _ _ _ _ _ _ _ _ _ _ _ _ _ _ _ _ _ _ _]
            tunnel: "Scan" -> [_ _ _ _ _ w503 w528 w542 w597 _ _ _ _ _ _ _ w698 _ _ _ _ _ _ _ _ _]
            tunnel: w190 -> [w221 _ w374 _ w483 w505 w530 w544 w599 _ w612 _ w635 w656 _ _ _ _ _ _ _ _ _ _ _ _]
            tunnel: w187 -> [w218 _ w373 _ _ _ _ _ _ _ _ _ _ _ _ _ _ _ _ _ _ _ _ _ _ _]
            tunnel: w189 -> [_ _ _ _ _ _ _ _ _ _ _ _ _ _ _ _ _ _ _ _ _ _ w763 w776 _ _]
            tunnel: w188 -> [_ _ _ _ _ _ w512 _ _ _ _ _ _ _ _ _ _ _ _ _ _ _ _ _ _ _]
            tunnel: w186 -> [w215 _ _ _ _ _ _ _ _ _ _ _ _ _ _ _ _ _ _ _ _ _ _ _ _ _]
            tunnel: w185 -> [w214 _ _ _ _ _ _ _ _ _ _ _ _ _ _ _ _ _ _ _ _ _ _ _ _ _]
            tunnel: w184 -> [w209 w349 w355 w472 w481 w502 w516 w540 w589 w607 w610 w619 w633 w653 w661 w693 w697 w724 w728 w732 w740 w749 w761 w773 w829 w849]
            tunnel: [w209 w349 w355 w472 w481 w501 w515 w538 w582 w607 w610 w619 w633 w653 w661 w693 w697 w724 w728 w732 w740 w749 w761 w773 w829 w849] -> w183
            tunnel: w182 -> [w208 w343 w352 w471 w480 w492 w514 w536 w577 w606 w609 w618 w632 w652 w658 w692 w696 w723 w727 w731 w739 w748 w760 w772 w825 w847]
            tunnel: [w208 w343 w351 w471 w480 w492 w513 w536 w579 w606 w609 w618 w632 w652 w658 w692 w695 w723 w727 w731 w739 w748 w759 w771 w828 w847] -> w181
            tunnel: w180 -> [w207 w348 w350 w470 w479 w499 w510 w535 w576 w604 w608 w617 w631 w651 w657 w691 w694 w722 w726 w730 w738 w747 w758 w770 w826 w846]
            tunnel: [w207 w348 w350 w470 w479 w497 w510 w535 w576 w604 w608 w617 w631 w651 w657 w691 w694 w722 w726 w730 w738 w747 w758 w770 w826 w846] -> w179
            event Timeout {
              n95 = event-data() -> ()  [unwired: 1 in, 1 out]
              n96 = Unbundle By Name(w221) -> ("DataBufferQ"=w220:refnum<queue>, "LastNQ"=w219:refnum<queue>)
              n97 = property class="VI"() -> (reference out=w216:refnum<vi>, "Front Panel.IsFrontmost"=w217:bool)  [unwired: 2 in, 1 out]
              n98 = Get Queue Status(queue=w220) -> (queue out=w225:refnum<queue>, error out=w224:errorcluster, # elements in queue=→"Image Backlog":i32)  [unwired: 2 in, 5 out]
              n99 = Dequeue Element(queue=w225, timeout in ms (-1)=250, error in (no error)=w224) -> (element=w212:T33, timed out?=w213:bool, error out=w222:errorcluster)  [unwired: 1 out]
              n100 = case shown="False" w217 {
                tunnel: w216 -> [w235 _]
                frame False {
                  n101 = property class="VI"(reference=w235, "Front Panel.IsFrontmost"=TRUE ("Front Panel Window:Is Frontmost")) -> ()  [unwired: 1 in, 2 out]
                }
                frame True {
                }
              }
              n102 = Unbundle(w212) -> ("Time Out"=w211:bool)  [unwired: 4 out]
              n103 = Or(x=w213, y=w211) -> (x .or. y?=w210:bool)
              "No data" <- w210
              n104 = case shown="False" w210 {
                tunnel: w229 -> [w262 _]
                tunnel: w219 -> [w277 _]
                tunnel: w234 -> [w276 _]
                tunnel: w212 -> [w275 _]
                tunnel: [w254 w329] -> w231
                tunnel: w230 -> [w267 w329]
                tunnel: w228 -> [w263 w328]
                tunnel: [w260 w328] -> w227
                tunnel: w226 -> [w258 _]
                tunnel: w218 -> [w255 _]
                tunnel: w222 -> [w250 _]
                tunnel: w215 -> [w246 _]
                tunnel: w214 -> [w244 _]
                tunnel: w209 -> [w243 _]
                tunnel: w208 -> [w242 _]
                tunnel: w207 -> [w241 _]
                frame False {
                  # "20log(abs(x) of binary values up to 25*2^7"
                  # "Get and display data"
                  n105 = flat-sequence {
                    tunnel: w250 -> [w297]
                    tunnel: [w297] -> w249
                    tunnel: [w296] -> w248
                    frame #0 {
                      n106 = Tick Count (ms)() -> (millisecond timer value=w296:u32)
                    }
                  }
                  n107 = Unbundle(w275) -> ("gain"=w268:dbl, w273:bool, "wfm"=w274:i16[][], "max queue size (-1, unlimited)"=→"Sat Ct":i32)  [unwired: 1 out]
                  n108 = case shown="True" w273 {
                    tunnel: w274 -> [w325 w327]
                    tunnel: [w325 w326] -> w257
                    tunnel: w249 -> [_ _]
                    frame False {
                    }
                    frame True {
                      n109 = call "ReverseData.vi"("Array in"=w327) -> ("Array out"=w326:i16[][])
                    }
                  }
                  n110 = Unbundle By Name(w241) -> ("GPU?"=w240:bool)
                  n111 = Not(x=w240) -> (.not. x?=w239:bool)
                  n112 = And(x="Filter", y=w239) -> (x .and. y?=w237:bool)
                  n113 = case shown="True" w237 {
                    tunnel: [w298 w301] -> w256
                    tunnel: w257 -> [w298 w300]
                    tunnel: w255 -> [_ w299]
                    frame False {
                    }
                    frame True {
                      n114 = call "BP FilterI16_Fast.vi"("Filter"=w299, "Array in"=w300) -> ("Filtered X"=w301:dbl[][])  [unwired: 4 in]
                    }
                  }
                  n115 = Bundle("gain"=w268, "Array out"=w257) -> (w269:cluster{"gain":dbl, "Array out":i16[][]})  [unwired: 1 in]
                  n116 = case shown="True" "Aviso Sector" {
                    tunnel: [w280 w289] -> w272
                    tunnel: w258 -> [w279 w288]
                    tunnel: w256 -> [w278 w295]
                    tunnel: w244 -> [_ w290]
                    frame False {
                      n117 = for {
                        tunnel: [w283] -> w280 mode=indexing
                        tunnel: w279 -> [w282]
                        tunnel: w278 -> [w281] mode=indexing
                        n118 = for {
                          tunnel: [w287] -> w283 mode=indexing
                          tunnel: w282 -> [w286]
                          tunnel: w281 -> [w285] mode=indexing
                          n119 = Absolute Value(x=w285) -> (abs(x)=w284:dbl)
                          n120 = Index Array(array=w286, index=w284) -> (element=w287:sgl)
                        }
                      }
                    }
                    frame True {
                      w294 = 0.0 ("X Scale.Offset and Multiplier:Offset")
                      n121 = Unbundle(w290) -> ("scales"=w291:cluster{"inc x (mm)":dbl, "inc y (mm)":dbl})  [unwired: 6 out]
                      n122 = call "AvisoSectorConvert.vi"("output cluster"=w290, "Log Lookup"=w288, "Raw In"=w295) -> ("Sector out"=w289:dbl[][])  [unwired: 8 in]
                      n123 = Unbundle(w291) -> ("inc x (mm)"=w293:dbl, "inc y (mm)"=w292:dbl)
                      n124 = property on="Raw data" class="IntGraph (strict)"("X Scale.Offset and Multiplier:Offset"=w294, "X Scale.Offset and Multiplier:Multiplier"=w293, "Y Scale.Offset and Multiplier:Offset"=w294, "Y Scale.Offset and Multiplier:Multiplier"=w292) -> ()  [unwired: 2 in, 2 out]
                    }
                  }
                  n125 = Lossy Enqueue Element(queue=w277, element=w269) -> (queue out=w266:refnum<queue>, error out=w264:errorcluster)  [unwired: 1 in, 2 out]
                  n126 = Get Queue Status(queue=w266, error in (no error)=w264) -> (# elements in queue=→"InQueue":i32)  [unwired: 1 in, 7 out]
                  n127 = case shown="True" "EYE CineLoop" {
                    tunnel: w257 -> [_ w324]
                    tunnel: w246 -> [_ w323]
                    tunnel: w262 -> [_ w316]
                    tunnel: w268 -> [_ w322]
                    tunnel: w276 -> [_ w321]
                    tunnel: w243 -> [_ w319]
                    tunnel: w242 -> [_ w318]
                    tunnel: w241 -> [_ w317]
                    frame False {
                    }
                    frame True {
                      n128 = Round Toward +Infinity(x=w323) -> (ceil(x): smallest int >= x=w320:dbl)
                      n129 = call "RT_Save_EYE.vi"("Data"=w324, "Eye Name"=w321, "Digitizer Gain"=w322, "Frame"=w316, "Digitizer Settings"=w319, "bits A/D"=w320, "Motion Settings"=w318, "Ann Array Params"=w317) -> ()  [unwired: 8 in]
                    }
                  }
                  n130 = case shown="True" "BMP CineLoop" {
                    tunnel: w262 -> [_ w313]
                    tunnel: w276 -> [_ w312]
                    frame False {
                    }
                    frame True {
                      n131 = invoke on="Raw data" class="IntGraph (strict)" method="Get Image"("image depth"=24) -> ("image data"=w314:T21)  [unwired: 5 in, 5 out]
                      n132 = call "RT_Save_JPG.vi"("Movie Name"=w312, "Frame"=w313, "image data"=w314) -> ()  [unwired: 9 in]
                    }
                  }
                  n133 = flat-sequence {
                    tunnel: w272 -> [w310]
                    tunnel: [w311] -> w254
                    frame #0 {
                      "Raw data" <- w310
                    }
                    frame #1 {
                      n134 = Tick Count (ms)() -> (millisecond timer value=w311:u32)
                    }
                  }
                  n135 = Greater?(x=w262, y=10) -> (0:w259:bool)
                  n136 = case shown="True" w259 {
                    tunnel: w267 -> [_ w307]
                    tunnel: w254 -> [_ w306]
                    tunnel: w263 -> [w302 w303]
                    tunnel: [w302 _] -> w260
                    frame False {
                    }
                    frame True {
                      n137 = Subtract(x=w306, y=w307) -> (x-y=w309:u32)
                      n138 = To Double Precision Float(number=w309) -> (double precision float=w308:dbl)
                      n139 = expression code="1000/x"(w308) -> (w305:dbl)
                      n140 = call <vilib>:"Mean PtByPt.vi"("x"=w305, "initialize"=w303) -> ("mean"=→"fps":dbl)  [unwired: 2 in, 1 out]
                    }
                  }
                  n141 = Subtract(x=w254, y=w248) -> (x-y=w252:u32)
                  n142 = call <vilib>:"Mean PtByPt.vi"("x"=w252, "sample length"=20) -> ("mean"=→"image time (ms)":dbl)  [unwired: 2 in, 1 out]
                  "Frame" <- w262
                }
                frame True {
                }
              }
            }
            event Key Down {
              n143 = event-data() -> ("VKey"=w346:T34, "Char"=w345:i16, "PlatMods"=w347:T35)  [unwired: 1 in]
              n144 = property on="Gate Length" class="DigNum (strict)"() -> ("Key Focus"=w342:bool)  [unwired: 2 in, 2 out]
              n145 = property on="Xtra delay (us)" class="DigNum (strict)"() -> ("Key Focus"=w340:bool)  [unwired: 2 in, 2 out]
              n146 = property on="LowTime" class="DigNum (strict)"() -> ("Key Focus"=w339:bool)  [unwired: 2 in, 2 out]
              n147 = property on="number of planes" class="DigNum (strict)"() -> ("Key Focus"=w338:bool)  [unwired: 2 in, 2 out]
              n148 = property on="Distance between\nplanes (mm)" class="DigNum (strict)"() -> ("Key Focus"=w337:bool)  [unwired: 2 in, 2 out]
              n149 = property on="RF data Sampling" class="Clust (strict)"() -> ("Key Focus"=w336:bool)  [unwired: 2 in, 2 out]
              n150 = property on="Filter Prams" class="Clust (strict)"() -> ("Key Focus"=w335:bool)  [unwired: 2 in, 2 out]
              n151 = property on="Inc. Step Size (mm)" class="DigNum (strict)"() -> ("Key Focus"=w334:bool)  [unwired: 2 in, 2 out]
              n152 = property on="Position (mm) (Abs)" class="DigNum (strict)"() -> ("Key Focus"=w333:bool)  [unwired: 2 in, 2 out]
              n153 = property on="File Name" class="Str"() -> ("Key Focus"=w332:bool)  [unwired: 2 in, 2 out]
              n154 = control-ref of="Position (mm) (Abs)"() -> (w330:refnum<vi>)
              n155 = control-ref of="Axis Tune"() -> (w331:refnum<vi>)
              n156 = Compound Arithmetic op=OR(w342, w340, w339, w338, w337, w336, w335, w334, w333, w332) -> (w341:bool)
              n157 = call "KeyboardNudge.vi"("Axis Tune Refnum"=w331, "Char"=w345, "Position (mm) Refnum"=w330, "Ignore Key Down"=w341, "VKey"=w346, "PlatMods"=w347, "Inc. Step Size (mm)"="Inc. Step Size (mm)", "Motion Settings"=w343) -> ()  [unwired: 10 in, 2 out]
            }
            event "3D Acq": Value Change {
              # "Take a 3D stack by pulling real-time images at set intevals"
              n158 = event-data() -> ()  [unwired: 1 in, 2 out]
              n159 = Unbundle By Name(w352) -> ("Motion Bd ID"=w353:u8, "Steps per mm"=w354:i32[])
              n160 = Unbundle By Name(w374) -> ("DataBufferQ"=w372:refnum<queue>)
              n161 = disable-structure shown="Disabled" {
                disable-tunnel: [w382 _] -> w370
                disable-tunnel: "Axis" -> [w381 _]
                disable-tunnel: [w380 _] -> w362
                disable-tunnel: [w379 _] -> w361
                disable-tunnel: w353 -> [w378 _]
                frame Disabled {
                  n162 = call <vilib>:"Read Position.flx"("Axis"=w381, "Board ID"=w378) -> ("Resource Output"=w379:T36, "Bd ID Out"=w380:T37, "Position"=w382:i32)  [unwired: 4 in, 1 out]
                }
                frame Enabled {
                }
              }
              n163 = call "NumberFileName.vi"("String"="", "Digits"=2, "File number"=w357, "file name"="") -> ("Numbered File"=w356:string)
              n164 = Decrement(x="Axis") -> (x-1=w369:u16)
              n165 = Index Array(array=w354, index=w369) -> (element=w363:i32)
              n166 = Multiply(x=0.001, y=w363) -> (x*y=w366:dbl)
              n167 = Multiply(x="Distance between\nplanes (mm)", y=w366) -> (x*y=w364:dbl)
              n168 = stacked-sequence {
                tunnel: w377 -> [_ w406 _]
                tunnel: w375 -> [_ w405 _]
                tunnel: w373 -> [_ w404 _]
                tunnel: w372 -> [_ w403 _]
                tunnel: "number of planes" -> [w392 w399 _]
                tunnel: w362 -> [w391 w402 w468]
                tunnel: w361 -> [w390 w401 w467]
                tunnel: w370 -> [_ _ w469]
                tunnel: "Distance between\nplanes (mm)" -> [w384 _ _]
                tunnel: w364 -> [w388 w400 _]
                tunnel: w356 -> [_ w398 _]
                tunnel: w355 -> [_ w397 _]
                tunnel: w352 -> [w385 w396 _]
                tunnel: [w383 _ _] -> w351
                tunnel: w350 -> [_ w395 _]
                frame #0 {
                  # "back up"
                  # "Move second axis to end and start scan"
                  n169 = Bundle By Name(cluster=w385, "Distance between\nscan planes (um)"=w384) -> (w383:T4)
                  n170 = Decrement(x=w392) -> (x-1=w393:u16)
                  n171 = Multiply(x=w393, y=w388) -> (x*y=w389:dbl)
                  n172 = Divide(x=w389, y=-2) -> (x/y=w386:dbl)
                  n173 = call "MoveMotor.vi"("Position Mode (Absolute)"=T23."Relative Position", "Target Position (0)"=w386, "Axis or Vector Space"=w390, "Motion Bd ID"=w391) -> ()  [unwired: 5 in, 3 out]
                }
                frame #1 {
                  n174 = for {
                    N: w399 -> [_]
                    tunnel: w406 -> [w418]
                    tunnel: w405 -> [w417]
                    tunnel: w404 -> [w416]
                    tunnel: w403 -> [w415]
                    tunnel: w402 -> [w414]
                    tunnel: w401 -> [w413]
                    tunnel: w400 -> [w411]
                    tunnel: w398 -> [w410]
                    tunnel: w397 -> [w409]
                    tunnel: w396 -> [w408]
                    tunnel: w395 -> [w407]
                    i -> [w412]
                    n175 = stacked-sequence {
                      tunnel: w418 -> [w431 _]
                      tunnel: w417 -> [w429 _]
                      tunnel: w416 -> [w425 _]
                      tunnel: w415 -> [w424 _]
                      tunnel: w414 -> [_ w466]
                      tunnel: w413 -> [_ w465]
                      tunnel: w412 -> [w423 _]
                      tunnel: w411 -> [_ w463]
                      tunnel: w410 -> [w422 _]
                      tunnel: w409 -> [w421 _]
                      tunnel: w408 -> [w420 _]
                      tunnel: w407 -> [w419 _]
                      frame #0 {
                        n176 = Dequeue Element(queue=w424, timeout in ms (-1)=2000) -> (element=w428:T33, timed out?=w427:bool, error out=w426:errorcluster)  [unwired: 1 in, 1 out]
                        n177 = case shown="False" w427 {
                          tunnel: w431 -> [w438 _]
                          tunnel: w428 -> [w452 _]
                          tunnel: w429 -> [w447 _]
                          tunnel: w425 -> [w436 _]
                          tunnel: w426 -> [w444 _]
                          tunnel: w423 -> [w432 _]
                          tunnel: w422 -> [w437 _]
                          tunnel: w421 -> [w435 _]
                          tunnel: w420 -> [w434 _]
                          tunnel: w419 -> [w433 _]
                          frame False {
                            # "20log(abs(x) of binary values up to 25*2^7"
                            # "Get and display data"
                            n178 = Unbundle(w452) -> ("gain"=w448:dbl, w450:bool, "wfm"=w451:i16[][])  [unwired: 2 out]
                            n179 = case shown="False" w450 {
                              tunnel: w451 -> [w460 w462]
                              tunnel: [w460 w461] -> w446
                              tunnel: w444 -> [_ _]
                              frame False {
                              }
                              frame True {
                                n180 = call "ReverseData.vi"("Array in"=w462) -> ("Array out"=w461:i16[][])
                              }
                            }
                            n181 = Concatenate Strings(w438, w437, "_3D" ("string")) -> (w440:string)
                            n182 = call "BP FilterI16_Fast.vi"("Filter"=w436, "Array in"=w446) -> ("Filtered X"=w445:dbl[][])  [unwired: 4 in]
                            n183 = local write "Frame"(w432) -> ()
                            n184 = invoke on="Raw data" class="IntGraph (strict)" method="Get Image"("image depth"=24) -> ("image data"=w441:T21)  [unwired: 5 in, 5 out]
                            n185 = call "RT_Save_EYE.vi"("Data"=w446, "Eye Name"=w440, "Digitizer Gain"=w448, "Frame"=w432, "Digitizer Settings"=w435, "bits A/D"=13, "Motion Settings"=w434, "Ann Array Params"=w433) -> ()  [unwired: 8 in]
                            n186 = for {
                              tunnel: [w455] -> w443 mode=indexing
                              tunnel: w447 -> [w454]
                              tunnel: w445 -> [w453] mode=indexing
                              n187 = for {
                                tunnel: [w459] -> w455 mode=indexing
                                tunnel: w454 -> [w458]
                                tunnel: w453 -> [w457] mode=indexing
                                n188 = Absolute Value(x=w457) -> (abs(x)=w456:dbl)
                                n189 = Index Array(array=w458, index=w456) -> (element=w459:sgl)
                              }
                            }
                            n190 = call "RT_Save_JPG.vi"("Movie Name"=w440, "Frame"=w432, "image data"=w441) -> ()  [unwired: 9 in]
                            n191 = local write "Raw data"(w443) -> ()
                          }
                          frame True {
                          }
                        }
                      }
                      frame #1 {
                        # "while loop until position is cross"
                        n192 = call "MoveMotor.vi"("Position Mode (Absolute)"=T23."Relative Position", "Target Position (0)"=w463, "Axis or Vector Space"=w465, "Motion Bd ID"=w466) -> ()  [unwired: 5 in, 3 out]
                      }
                    }
                  }
                }
                frame #2 {
                  # "Return to start"
                  n193 = call "MoveMotor.vi"("Target Position (0)"=w469, "Axis or Vector Space"=w467, "Motion Bd ID"=w468) -> ()  [unwired: 6 in, 3 out]
                }
              }
            }
            event "number of planes", "Distance between\nplanes (mm)": Value Change {
              n194 = event-data() -> ()  [unwired: 1 in, 5 out]
              n195 = local read "Distance between\nplanes (mm)"() -> (w476:i32)
              n196 = local read "number of planes"() -> (w478:u16)
              n197 = Decrement(x=w478) -> (x-1=w477:u16)
              n198 = Multiply(x=w477, y=w476) -> (x*y=w475:i32)
              n199 = Multiply(x=w475, y=sgl 0.001) -> (x*y=→"Length of\nall planes (cm)":sgl)
            }
            event "Scan": Value Change {
              n200 = event-data() -> ("NewVal"=w485:bool)  [unwired: 1 in, 4 out]
              n201 = Unbundle By Name(w483) -> ("StopN"=w482:refnum<notifier>)
              n202 = case shown="False" w485 {
                selector: w485 -> [w486 w491]
                tunnel: [w486 w491] -> w484
                tunnel: w482 -> [w487 _]
                frame False {
                  n203 = flat-sequence {
                    tunnel: w487 -> [w488]
                    frame #0 {
                      n204 = Send Notification(notification=TRUE, notifier=w488) -> ()  [unwired: 1 in, 2 out]
                    }
                    frame #1 {
                      n205 = Wait (ms)(milliseconds to wait=u32 500) -> ()  [unwired: 1 out]
                    }
                  }
                }
                frame True {
                }
              }
            }
            event "Xtra delay (us)", "Focal Zones", "Filter Prams", "Pause", "GPU?", "Xmt/Rcv": Value Change {
              n206 = event-data() -> ()  [unwired: 1 in, 1 out]
              n207 = Bundle By Name(cluster=w502, "Xtra Ann Trig delay (us)"="Xtra delay (us)") -> (w501:T8)
              n208 = call "F-Zones.vi"("Trans Geometry (mm)"="Trans Geometry (mm)") -> ("Trans Geometry (mm) out"=w495:T2)  [unwired: 7 in, 3 out]
              n209 = Unbundle By Name(w505) -> ("StopN"=w504:refnum<notifier>)
              n210 = local write "Trans Geometry (mm)"(w495) -> ()
              n211 = case shown="True" w503 {
                tunnel: w504 -> [_ w506]
                frame False {
                }
                frame True {
                  n212 = flat-sequence {
                    tunnel: w506 -> [w507]
                    frame #0 {
                      n213 = Send Notification(notification=TRUE, notifier=w507) -> ()  [unwired: 1 in, 2 out]
                    }
                    frame #1 {
                      n214 = Wait (ms)(milliseconds to wait=u32 500) -> ()  [unwired: 1 out]
                    }
                  }
                }
              }
              n215 = Bundle By Name(cluster=w499, "Trans Geometry (mm)"=w495, "Focal Zones"="Focal Zones", "Xmt/Rcv"="Xmt/Rcv", "GPU?"="GPU?") -> (w497:T1)
            }
            event "Motion Parameters": Value Change {
              n216 = event-data() -> ("NewVal"=w517:T15)  [unwired: 1 in]
              n217 = Unbundle By Name(w517) -> ("lines per plane"=w511:u16, "Overshoot"=w518:i32, "BKPT Shift"=w527:i32, "Frames/s"=w526:sgl, "Distance between\nscan lines (um)"=w522:sgl)
              n218 = Unbundle By Name(w514) -> ("Steps per mm"=w524:i32[])
              n219 = Unbundle By Name(w530) -> ("StopN"=w529:refnum<notifier>)
              n220 = Decrement(x=w512) -> (x-1=w525:T18)
              n221 = case shown="True" w528 {
                tunnel: w529 -> [_ w531]
                frame False {
                }
                frame True {
                  n222 = flat-sequence {
                    tunnel: w531 -> [w532]
                    frame #0 {
                      n223 = Send Notification(notification=TRUE, notifier=w532) -> ()  [unwired: 1 in, 2 out]
                    }
                    frame #1 {
                      n224 = Wait (ms)(milliseconds to wait=u32 500) -> ()  [unwired: 1 out]
                    }
                  }
                }
              }
              n225 = Index Array(array=w524, index=w525) -> (element=w521:i32)
              n226 = Decrement(x=w511) -> (x-1=w523:u16)
              n227 = Bundle By Name(cluster=w516, "lines per plane"=w511) -> (w515:T8)
              n228 = Compound Arithmetic op=MULTIPLY(w523, w522, w521, 0.001) -> (w519:dbl)
              n229 = Bundle By Name(cluster=w514, "overshoot cts"=w518, "BKPT Shift"=w527, "RT fps"=w526, "Distance between\nscan lines (um)"=w522, "Total steps in line"=w519) -> (w513:T4)
            }
            event "Voltage": Value Change {
              n230 = event-data() -> ("NewVal"=w539:dbl)  [unwired: 1 in]
              n231 = Unbundle By Name(w544) -> ("StopN"=w543:refnum<notifier>)
              n232 = case shown="True" w542 {
                tunnel: w543 -> [_ w570]
                tunnel: [_ w568] -> w541
                frame False {
                }
                frame True {
                  n233 = flat-sequence {
                    tunnel: w570 -> [w572]
                    tunnel: [w571] -> w569
                    tunnel: w569 -> [w574]
                    tunnel: [w574] -> w568
                    frame #0 {
                      n234 = Send Notification(notification=TRUE, notifier=w572) -> (error out=w571:errorcluster)  [unwired: 1 in, 1 out]
                    }
                    frame #1 {
                      n235 = Wait (ms)(milliseconds to wait=u32 500) -> ()  [unwired: 1 out]
                    }
                  }
                }
              }
              n236 = Bundle By Name(cluster=w540, "Voltage Scale"=w539) -> (w538:T8)
              n237 = Unbundle By Name(w538) -> ("Main Digitizer"=w537:T9)
              n238 = case shown="\"AlazarTech\"" w537 {
                tunnel: w538 -> [w546 w559]
                tunnel: w541 -> [w548 _]
                tunnel: w539 -> [w547 w557]
                frame "NI Digitizer", Default {
                  n239 = Unbundle By Name(w546) -> ("Digitizer ID Cluster.NI Instr Handles"=w545:refnum<k15>[])
                  n240 = for {
                    tunnel: w545 -> [w552] mode=indexing
                    tunnel: w547 -> [w550]
                    tunnel: w548 -> [w549]
                    n241 = property class="niScope"(reference=w552, error in=w549, "Active Channel"="0,1", "Vertical Range"=w550) -> ()  [unwired: 2 out]
                  }
                }
                frame "AlazarTech" {
                  n242 = Unbundle By Name(w559) -> ("Digitizer ID Cluster.Acqiris/Alazar/SP ID"=w553:u32[])
                  n243 = Array Size(array=w553) -> (size(s)=w555:i32)
                  n244 = case shown="2" w555 {
                    tunnel: [w560 w561] -> w554
                    frame 2 {
                      w560 = u8[] [1, 2] items=["A"=1, "B"=2, "C"=4, "D"=8]
                    }
                    frame 1, Default {
                      w561 = u8[] [1, 2, 4, 8] items=["A"=1, "B"=2, "C"=4, "D"=8]
                    }
                  }
                  n245 = Bundle By Name(cluster=T24 {"Voltage Scale"=0.0, "Offset"=0.0, "Coupling"=2} ("V scale"), "Voltage Scale"=w557) -> (w556:T24)
                  n246 = for {
                    tunnel: w553 -> [w564] mode=indexing
                    tunnel: w556 -> [w563]
                    tunnel: w554 -> [w562]
                    n247 = for {
                      tunnel: w564 -> [w566]
                      tunnel: w563 -> [w567]
                      tunnel: w562 -> [w565] mode=indexing
                      n248 = call "Alazar_ChannelConfig - ATS-SDK.vi"("V scale"=w567, "Channel"=w565, "Handle in"=w566) -> ()  [unwired: 2 in, 3 out]
                    }
                  }
                }
              }
            }
            event "RF data Sampling": Value Change {
              n249 = event-data() -> ("NewVal"=w594:T14)  [unwired: 1 in]
              n250 = Unbundle By Name(w599) -> ("StopN"=w598:refnum<notifier>)
              n251 = Unbundle(w594) -> ("Sampling Rate"=w595:dbl, "Ref Delay (ms)"=w592:dbl, "rf points per line"=w591:i32)
              n252 = expression code="x*1E6"(w595) -> (w593:dbl)
              n253 = case shown="False" w597 {
                tunnel: w598 -> [_ w600]
                frame False {
                }
                frame True {
                  n254 = flat-sequence {
                    tunnel: w600 -> [w601]
                    frame #0 {
                      n255 = Send Notification(notification=TRUE, notifier=w601) -> ()  [unwired: 1 in, 2 out]
                    }
                    frame #1 {
                      n256 = Wait (ms)(milliseconds to wait=u32 500) -> ()  [unwired: 1 out]
                    }
                  }
                }
              }
              n257 = Bundle By Name(cluster=w589, "rf points per line"=w591, "Digitizer delay (us)"=w592, "Samp Rate (Hz)"=w593) -> (w582:T8)
              n258 = Unbundle By Name(w577) -> ("Distance between\nscan lines (um)"=w581:sgl)
              n259 = Unbundle By Name(w582) -> ("lines per plane"=w590:i32)
              n260 = call "PlotScalingParams.vi"("Motion Settings In"=w577, "c mm/mics"=sgl 1.485, "Digitizer Settings"=w582, "Scan Axis"=w583) -> ("Cluster"=w588:T38)  [unwired: 5 in, 2 out]
              n261 = Decrement(x=w590) -> (x-1=w596:i32)
              n262 = Multiply(x=w596, y=w581) -> (x*y=w580:sgl)
              n263 = Bundle By Name(cluster=w577, "Total steps in line"=w580) -> (w579:T4)
              n264 = Unbundle By Name(w588) -> ("X Scale Offset"=w587:dbl, "X Scale Multi"=w586:dbl, "Y Scale Offset"=w585:dbl, "Y Scale Multi"=w584:dbl)
              n265 = property on="Raw data" class="IntGraph (strict)"("X Scale.Offset and Multiplier:Offset"=w587, "X Scale.Offset and Multiplier:Multiplier"=w586, "Y Scale.Offset and Multiplier:Offset"=w585, "Y Scale.Offset and Multiplier:Multiplier"=w584) -> ()  [unwired: 2 in, 2 out]
            }
            event "Daxsonics Settings": Value Change {
              n266 = event-data() -> ("NewVal"=w605:T13)  [unwired: 1 in]
              n267 = call "Set_Daxsonics_3Pulsers.vi"("Daxsonics Settings"=w605) -> ()  [unwired: 9 in]
            }
            event "ExitSendCmd": Value Change {
              n268 = event-data() -> ()  [unwired: 1 in, 5 out]
              n269 = Unbundle By Name(w612) -> ("StopN"=w611:refnum<notifier>)
              n270 = flat-sequence {
                tunnel: w611 -> [w614]
                frame #0 {
                  n271 = Send Notification(notification=TRUE, notifier=w614) -> ()  [unwired: 1 in, 2 out]
                }
                frame #1 {
                  n272 = Wait (ms)(milliseconds to wait=u32 500) -> ()  [unwired: 1 out]
                }
              }
            }
            event "File Name": Value Change {
              # "Pull all named files"
              n273 = event-data() -> ("NewVal"=w622:string)  [unwired: 1 in]
              n274 = global read "MotionGlobals.vi" "TempPath"() -> (w621:path)
              n275 = Concatenate Strings(w622, "*") -> (w629:string)
              n276 = List Folder(path=w621, pattern=w629) -> (filenames=w627:string[])  [unwired: 1 in, 4 out]
              n277 = global read "MotionGlobals.vi" "SavePath"() -> (w620:path)
              n278 = List Folder(path=w620, pattern=w629) -> (filenames=w628:string[])  [unwired: 1 in, 4 out]
              n279 = Array Size(array=w627) -> (size(s)=w625:i32)
              n280 = Array Size(array=w628) -> (size(s)=w626:i32)
              n281 = Add(x=w626, y=w625) -> (x+y=w624:i32)
              n282 = case shown="0" w624 {
                frame 0 {
                }
                frame 1, Default {
                  n283 = One Button Dialog(message="File name has been used already. Select a new file name.") -> ()  [unwired: 1 in, 1 out]
                }
              }
            }
            event "Save Last N EYE": Value Change {
              n284 = event-data() -> ()  [unwired: 1 in, 5 out]
              n285 = Unbundle By Name(w635) -> ("LastNQ"=w634:refnum<queue>)
              n286 = Flush Queue(queue=w634) -> (remaining elements=w637:cluster{"gain":dbl, "wfm":i16[][]}[])  [unwired: 1 in, 2 out]
              n287 = for {
                N: "N" -> [_]
                tunnel: w639 -> [w648]
                tunnel: w638 -> [w645]
                tunnel: w637 -> [w644] mode=indexing
                tunnel: w633 -> [w643]
                tunnel: w632 -> [w642]
                tunnel: w631 -> [w641]
                i -> [w647]
                n288 = Unbundle(w644) -> ("gain"=w649:dbl, "wfm"=w646:i16[][])
                n289 = Subtract(x=w648, y=w647) -> (x-y=w640:i32)
                n290 = call "RT_Save_EYE.vi"("Data"=w646, "Eye Name"=w645, "Digitizer Gain"=w649, "Frame"=w640, "Digitizer Settings"=w643, "bits A/D"=11, "Motion Settings"=w642, "Ann Array Params"=w641) -> ()  [unwired: 8 in]
              }
            }
            event "Save Raw": Value Change {
              n291 = event-data() -> ()  [unwired: 1 in, 5 out]
              n292 = Unbundle By Name(w656) -> ("SaveRawN"=w654:refnum<notifier>)
              n293 = Send Notification(notification="Save Raw", notifier=w654) -> ()  [unwired: 1 in, 2 out]
            }
            event "1-to-1": Value Change {
              n294 = event-data() -> ()  [unwired: 1 in, 5 out]
              n295 = Unbundle By Name(w661) -> ("lines per plane"=w660:i32, "rf points per line"=w659:i32)
              n296 = property on="Raw data" class="IntGraph (strict)"() -> ("X Scale.Offset and Multiplier:Multiplier"=w675:dbl, "Y Scale.Offset and Multiplier:Multiplier"=w674:dbl)  [unwired: 2 in, 2 out]
              n297 = Multiply(x=w660, y=w675) -> (x*y=w673:dbl)
              n298 = Multiply(x=w674, y=w659) -> (x*y=w672:dbl)
              n299 = Unbundle(w663) -> ("Width"=w667:u32, "Height"=w665:u32)
              n300 = Divide(x=w667, y=w673) -> (x/y=w671:dbl)
              n301 = Divide(x=w665, y=w672) -> (x/y=w670:dbl)
              n302 = Divide(x=w671, y=w670) -> (x/y=w666:dbl)
              n303 = Greater?(x=w666, y=1.0) -> (0:w669:bool)
              n304 = case shown="False" w669 {
                tunnel: w667 -> [_ w689]
                tunnel: w666 -> [w682 w688]
                tunnel: w665 -> [w681 _]
                tunnel: w662 -> [w676 w687]
                tunnel: [w677 w683] -> w664
                frame False {
                  n305 = Unbundle By Name(w676) -> ("Top"=w680:i16)
                  n306 = Multiply(x=w681, y=w682) -> (x*y=w678:dbl)
                  n307 = Add(x=w680, y=w678) -> (x+y=w679:dbl)
                  n308 = Bundle By Name(cluster=w676, "Bottom"=w679) -> (w677:T17)
                }
                frame True {
                  n309 = Unbundle By Name(w687) -> ("Left"=w685:i16)
                  n310 = Divide(x=w689, y=w688) -> (x/y=w686:dbl)
                  n311 = Add(x=w685, y=w686) -> (x+y=w684:dbl)
                  n312 = Bundle By Name(cluster=w687, "Right"=w684) -> (w683:T17)
                }
              }
              n313 = property on="Raw data" class="IntGraph (strict)"("Plot Bounds"=w664) -> ()  [unwired: 2 in, 2 out]
            }
            event "Flip X": Value Change {
              n314 = event-data() -> ()  [unwired: 1 in, 6 out]
              n315 = property on="Raw data" class="IntGraph (strict)"("XScale.Flipped"="Flip X") -> ()  [unwired: 2 in, 2 out]
            }
            event "Center": Value Change {
              n316 = event-data() -> ()  [unwired: 1 in, 5 out]
              n317 = case shown="False" w698 {
                tunnel: w699 -> [w704 _]
                tunnel: w696 -> [w701 w721]
                tunnel: [w702 w721] -> w695
                frame False {
                  n318 = Unbundle By Name(w701) -> ("Motion System"=w700:T5)
                  n319 = case shown="\"NI 735x\"" w700 {
                    tunnel: w704 -> [_ w707 w718]
                    tunnel: [_ w706 w716] -> w703
                    tunnel: w701 -> [_ w705 w720]
                    frame "MM3000", Default {
                    }
                    frame "NI 735x" {
                      n320 = disable-structure shown="Disabled" {
                        disable-tunnel: w707 -> [w711 _]
                        disable-tunnel: [w710 _] -> w706
                        disable-tunnel: w705 -> [w708 _]
                        frame Disabled {
                          n321 = Unbundle By Name(w708) -> ("Motion Bd ID"=w709:u8)
                          n322 = call <vilib>:"Find Reference.flx"("Search Type"=T25."Center", "Axis or Vector Space"=w711, "Board ID"=w709) -> ("error out"=w714:errorcluster, "Axis or Vector Space Output"=w713:T39, "Bd ID Out"=w712:T37)  [unwired: 6 in]
                          n323 = call <vilib>:"Wait Reference.flx"("error in (no error)"=w714, "Axis or Vector Space"=w713, "Board ID"=w712) -> ("error out"=w710:errorcluster)  [unwired: 5 in, 3 out]
                        }
                        frame Enabled {
                        }
                      }
                    }
                    frame "Galil" {
                      n324 = Unbundle By Name(w720) -> ("GL Ref Out"=w719:refnum<k7>)
                      n325 = Decrement(x=w718) -> (x-1=w717:i32)
                      n326 = call "GL Center.vi"("Axis"=w717, "Galil.IGalil"=w719) -> ("error out"=w716:errorcluster)  [unwired: 5 in, 2 out]
                    }
                  }
                  n327 = call "FindLocation.vi"("Motion Settings"=w701, "error in (no error)"=w703) -> ("Motion Settings Out"=w702:T4)  [unwired: 1 in, 3 out]
                }
                frame True {
                }
              }
            }
            event "Fill": Value Change {
              n328 = event-data() -> ()  [unwired: 1 in, 5 out]
              n329 = property on="Raw data" class="IntGraph (strict)"("Plot Bounds"=w725) -> ()  [unwired: 2 in, 2 out]
            }
            event "Auto\nScale": Value Change {
              w729 = u8 1 ("X Scale.Scale Fit")
              n330 = event-data() -> ()  [unwired: 1 in, 5 out]
              n331 = property on="Raw data" class="IntGraph (strict)"("XScale.ScaleFit"=w729, "YScale.ScaleFit"=w729) -> ()  [unwired: 2 in, 2 out]
            }
            event "Scale (dB)": Value Change {
              n332 = event-data() -> ("NewVal"=w737:cluster{i32, i32})  [unwired: 1 in, 4 out]
              n333 = Unbundle(w737) -> (w735:i32, w734:i32)
              n334 = property on="Raw data" class="IntGraph (strict)"() -> ("ZScale.Range"=w736:T40)  [unwired: 2 in, 2 out]
              n335 = Bundle By Name(cluster=w736, "Minimum"=w734, "Maximum"=w735) -> (w733:T40)
              n336 = property on="Raw data" class="IntGraph (strict)"("ZScale.Range"=w733) -> ()  [unwired: 2 in, 2 out]
            }
            event "Adjust fps (%)": Value Change {
              n337 = event-data() -> ()  [unwired: 1 in, 5 out]
              n338 = disable-structure shown="Disabled" {
                disable-tunnel: "Adjust fps (%)" -> [w746 _]
                disable-tunnel: w741 -> [w745 _]
                disable-tunnel: w739 -> [w744 _]
                frame Disabled {
                  n339 = Unbundle By Name(w744) -> ("Motion Bd ID"=w743:u8)
                  n340 = call <vilib>:"Load Velocity Override.flx"("Override  Percentage (100%)"=w746, "Axis or Vector Space"=w745, "Board ID"=w743) -> ()  [unwired: 4 in, 3 out]
                }
                frame Enabled {
                }
              }
            }
            event "Accel": Value Change {
              n341 = event-data() -> ("NewVal"=w751:dbl)  [unwired: 1 in]
              n342 = disable-structure shown="Disabled" {
                disable-tunnel: w752 -> [w757 _]
                disable-tunnel: w751 -> [w756 _]
                disable-tunnel: enum16{"Both", "Acceleration", "Deceleration"}."Acceleration" ("Acceleration Type (Both)") -> [w755 _]
                disable-tunnel: w748 -> [w754 _]
                frame Disabled {
                  n343 = Unbundle By Name(w754) -> ("Motion Bd ID"=w753:u8)
                  n344 = call "Load Acceleration/Deceleration.flx"("Acceleration Type (Both)"=w755, "Acceleration (100000)"=w756, "Axis or Vector Space"=w757, "Board ID"=w753) -> ()  [unwired: 3 in, 3 out]
                }
                frame Enabled {
                }
              }
            }
            event "Axis Tune": Value Change {
              n345 = event-data() -> ("NewVal"=w762:enum32{"Axis 1", "Axis 2", "Axis 3", "Axis 4"})  [unwired: 1 in]
              n346 = case shown="\"MM3000\", \"Newport ESP\", \"No Motion Card\"" w763 {
                tunnel: w762 -> [w768 _]
                tunnel: w760 -> [w764 w769]
                tunnel: [w765 w769] -> w759
                frame "NI 735x", Default {
                  n347 = call "FindLocation_SingleAxis.vi"("Axis (0 is X)"=w768, "Motion Settings"=w764) -> ("Global Position"=w766:dbl[], "Position (mm) (Abs)"=w767:dbl)  [unwired: 2 in, 2 out]
                  n348 = local write "Position (mm) (Abs)"(w767) -> ()
                  n349 = Bundle By Name(cluster=w764, "Global Position (mm)"=w766) -> (w765:T4)
                }
                frame "MM3000", "Newport ESP", "No Motion Card" {
                }
              }
            }
            event "Position (mm) (Abs)": Value Change {
              n350 = event-data() -> ("NewVal"=w774:dbl)  [unwired: 1 in]
              n351 = case shown="\"NI 735x\", Default" w776 {
                tunnel: w775 -> [_ w786]
                tunnel: w774 -> [_ w783]
                tunnel: w772 -> [w777 w781]
                tunnel: [w777 w779] -> w771
                frame "MM3000", "Newport ESP", "No Motion Card" {
                }
                frame "NI 735x", Default {
                  n352 = Unbundle By Name(w781) -> ("Steps per mm"=w780:i32[])
                  n353 = local read "Axis Tune"() -> (w784:enum32{"Axis 1", "Axis 2", "Axis 3", "Axis 4"})
                  n354 = Index Array(array=w780, index=w784) -> (element=w790:i32)
                  n355 = Decrement(x=w786) -> (x-1=w782:i32)
                  n356 = Equal?(x=w784, y=w782) -> (x = y?=w785:bool)
                  n357 = To Byte Integer(number=w784) -> (8bit integer=w787:i8)
                  n358 = Multiply(x=w783, y=w790) -> (x*y=w789:dbl)
                  n359 = Increment(x=w787) -> (x+1=w778:i8)
                  n360 = case shown="\"Axis 3\"" w784 {
                    tunnel: w789 -> [w818 w822]
                    tunnel: [w818 w821] -> w788
                    tunnel: w781 -> [_ w820]
                    frame "Axis 1", Default {
                    }
                    frame "Axis 3" {
                      n361 = Unbundle By Name(w820) -> ("Reverse Z axis?"=w819:bool)
                      n362 = Negate(x=w822) -> (-x=w823:dbl)
                      n363 = Select(t=w823, s=w819, f=w822) -> (s? t:f=w821:dbl)
                    }
                  }
                  n364 = case shown="False" w785 {
                    tunnel: w778 -> [w794 _]
                    tunnel: w788 -> [w793 _]
                    tunnel: w784 -> [_ w816]
                    tunnel: w781 -> [w792 w815]
                    tunnel: [w792 w813] -> w779
                    frame False {
                      n365 = Unbundle By Name(w792) -> ("Motion System"=w791:T5)
                      n366 = case shown="\"NI 735x\"" w791 {
                        tunnel: w794 -> [_ w797 w810]
                        tunnel: w793 -> [_ w796 w808]
                        tunnel: w792 -> [_ w795 w812]
                        frame "MM3000", Default {
                        }
                        frame "NI 735x" {
                          n367 = disable-structure shown="Disabled" {
                            disable-tunnel: w797 -> [w807 _]
                            disable-tunnel: w796 -> [w800 _]
                            disable-tunnel: w795 -> [w798 _]
                            frame Disabled {
                              n368 = Unbundle By Name(w798) -> ("Motion Bd ID"=w799:u8)
                              n369 = call <vilib>:"Set Operation Mode.flx"("Axis or Vector Space"=w807, "Board ID"=w799) -> ("error out"=w806:errorcluster, "Resource Output"=w804:T36, "Bd ID Out"=w805:T37)  [unwired: 4 in]
                              n370 = call <vilib>:"Load Target Position.flx"("Target Position (0)"=w800, "error in (no error)"=w806, "Axis"=w804, "Board ID"=w805) -> ("error out"=w802:errorcluster, "Resource Output"=w801:T36, "Bd ID Out"=w803:T37)  [unwired: 3 in]
                              n371 = call-poly <vilib>:"Start Motion.flx"("error in (no error)"=w802, "Axis or Vector Space"=w801, "Board ID"=w803) -> ()  [unwired: 3 in, 3 out]
                            }
                            frame Enabled {
                            }
                          }
                        }
                        frame "Galil" {
                          n372 = Unbundle By Name(w812) -> ("GL Ref Out"=w811:refnum<k7>)
                          n373 = Decrement(x=w810) -> (x-1=w809:i8)
                          n374 = call "GL Set Operation Mode.vi"("position cts (abs/rel)"=w808, "Axis"=w809, "Galil.IGalil"=w811) -> ()  [unwired: 6 in, 3 out]
                        }
                      }
                    }
                    frame True {
                      n375 = call "FindLocation_SingleAxis.vi"("Axis (0 is X)"=w816, "Motion Settings"=w815) -> ("Global Position"=w814:dbl[], "Position (mm) (Abs)"=w817:dbl)  [unwired: 2 in, 2 out]
                      n376 = Bundle By Name(cluster=w815, "Global Position (mm)"=w814) -> (w813:T4)
                      n377 = local write "Position (mm) (Abs)"(w817) -> ()
                    }
                  }
                }
              }
            }
            event "Stop Motor": Value Change {
              n378 = event-data() -> ()  [unwired: 1 in, 1 out]
              n379 = local read "Axis Tune"() -> (w832:enum32{"Axis 1", "Axis 2", "Axis 3", "Axis 4"})
              n380 = Unbundle By Name(w825) -> ("Motion System"=w824:T5)
              n381 = case shown="\"NI 735x\"" w824 {
                tunnel: w832 -> [_ w835 _]
                tunnel: [_ w834 w842] -> w830
                tunnel: w825 -> [_ w833 w845]
                frame "MM3000", Default {
                }
                frame "NI 735x" {
                  n382 = disable-structure shown="Disabled" {
                    disable-tunnel: w835 -> [w839 _]
                    disable-tunnel: [w838 _] -> w834
                    disable-tunnel: w833 -> [w836 _]
                    frame Disabled {
                      n383 = Unbundle By Name(w836) -> ("Motion Bd ID"=w837:u8)
                      n384 = Increment(x=w839) -> (x+1=w840:enum32{"Axis 1", "Axis 2", "Axis 3", "Axis 4"})
                      n385 = call-poly <vilib>:"Stop Motion.flx"("Stop Type (Decel)"=enum16{"Decelerate", "Halt", "Kill"}."Halt", "Axis or Vector Space"=w840, "Board ID"=w837) -> ("error out"=w838:errorcluster)  [unwired: 4 in, 2 out]
                    }
                    frame Enabled {
                    }
                  }
                }
                frame "Galil" {
                  n386 = Unbundle By Name(w845) -> ("GL Ref Out"=w843:refnum<k7>)
                  n387 = call "GL Command Set.vi"("Command"=Command_Menu."Abort Motion", "Galil.IGalil"=w843) -> ("error out"=w842:errorcluster)  [unwired: 5 in, 4 out]
                }
              }
              n388 = call "FindLocation_SingleAxis.vi"("error in (no error)"=w830, "Axis (0 is X)"=w832, "Motion Settings"=w825) -> ("Global Position"=w827:dbl[], "Position (mm) (Abs)"=w831:dbl)  [unwired: 1 in, 2 out]
              n389 = local write "Position (mm) (Abs)"(w831) -> ()
              n390 = Bundle By Name(cluster=w825, "Global Position (mm)"=w827) -> (w828:T4)
            }
            event "Gate Length", "LowTime": Value Change {
              n391 = event-data() -> ()  [unwired: 1 in, 4 out]
              n392 = Unbundle By Name(w849) -> ("Main Digitizer"=w848:T9)
              n393 = call "FrameSync.vi"("LowTime"="LowTime", "Gate Length"="Gate Length", "Main Digitizer"=w848) -> ()  [unwired: 7 in, 2 out]
            }
          }
          n394 = Or(x=w202, y=w200) -> (x .or. y?=w201:bool)
        }
      }
      "Digitizer Settings Out" <- w108
      "Motion Settings Out" <- w106
      "Ann Array\nParams Out" <- w105
    }
    frame #3 {
      w852 = TRUE ("force destroy? (F)")
      n395 = Unbundle By Name(w857) -> ("DataBufferQ"=w856:refnum<queue>, "StopN"=w855:refnum<notifier>, "LastNQ"=w854:refnum<queue>, "LastNBMPQ"=w853:refnum<queue>)
      n396 = local write "Scan"(FALSE ("go")) -> ()
      n397 = Release Queue(queue=w854, force destroy? (F)=w852) -> ()  [unwired: 1 in, 3 out]
      n398 = Release Notifier(notifier=w855, force destroy? (F)=w852) -> ()  [unwired: 1 in, 3 out]
      n399 = Release Queue(queue=w856, force destroy? (F)=w852) -> ()  [unwired: 1 in, 3 out]
      n400 = Release Queue(queue=w853, force destroy? (F)=w852) -> ()  [unwired: 1 in, 3 out]
    }
  }
